vi "Parse Downlink.vi"(7 "CP_DATA IN":u8[](array[numeric]), 8 "error in (no error)":errorcluster, 9 "Parameters":string, 10 "EXID":u32 step=1 format="%06x", 11 "Command":T1) -> (0 "error out":errorcluster, 2 "Downlink":u8[][](array[numeric]) format="%02x")   [LabVIEW 2020]
uses:
  Command List.ctl
  Typedef Command List.ctl
  <vilib>/Utility/miscctls.llb/LVDateTimeRec.ctl
panel:
  in  "Command":T2 items=["Get xPG Status", "xPG Stimulation", "Select Program", "Increment Program Amplitude", "Decrement Program Amplitude", "Get PoP Constants", "Get PPC Constants", "Get Program Names", "Set Pulse Amplitude", "Increment Pulse Amplitude", "Decrement Pulse Amplitude", "Get Pulse Widths", "Set Pulse Widths", "Increment Pulse Width", "Decrement Pulse Width", "Get Program Frequency", "Set Program Frequency", "Increment Program Frequency", "Decrement Program Frequency", "reserved", "Charging Control", "Get xPG Identity", "Set xPG Identity", "Restore Program Defaults", "Get Program Definition", "Set Program Definition", "Get Program Constants", "Set Program Constants", "Get Configurable Device Parameters", "Set Configurable Device Parameters", "Get Pulse Constants", "Set Pulse Constants", "Get Lead Limits", "Set Lead Limits", "Get Channel Calibrations", "Set Channel Calibrations", "reserved", "reserved", "reserved", "reserved", "reserved", "reserved", "Get Stim Asic HV Calibrations", "Set Stim Asic HV Calibrations", "reserved", "reserved", "Get CP Data", "Set CP Data", "Clear Log", "Read Log", "Append Log", "Get Patient Program Runtime", "Set Patient Program Runtimec", "Impedance Measurement", "Enter Storage Mode", "Echo Short", "Echo Long", "Get General Calibration", "Set General Calibration", "Get Trim List", "Set Trim List", "Get Counter", "Set Counter", "Get Test Stimulation", "Set Test Stimulation", "Get Titration Stimulation", "Set Titration Stimulation", "Get Ramp Time", "Set Ramp Time", "Get VBAT", "Set Software Description Block", "Write Memory", "Read Memory", "Reset xPG", "Erase Flash Block", "Write Vectors", "Read Vectors", "Diagnostic Data", "Set Background Impedance", "Get Background Impedence ", "Undefined"]
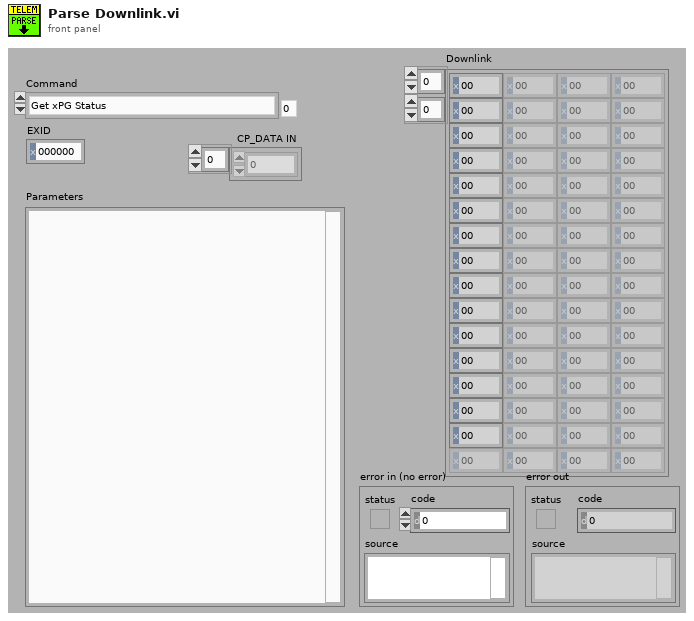
[diagram p1: front panel]
types:
  T1 = typedef "Typedef Command List.ctl" = enum16{"Get xPG Status", "xPG Stimulation", "Select Program", "Increment Program Amplitude", "Decrement Program Amplitude", "Get PoP Constants", "Get PPC Constants", "Get Program Names", "Set Pulse Amplitude", "Increment Pulse Amplitude", "Decrement Pulse Amplitude", "Get Pulse Widths", "Set Pulse Widths", "Increment Pulse Width", "Decrement Pulse Width", "Get Program Frequency", "Set Program Frequency", "Increment Program Frequency", "Decrement Program Frequency", "Inject Event", "Charging Control", "Get xPG Identity", "Set xPG Identity", "Restore Program Defaults", "Get Program Definition", "Set Program Definition", "Get Program Constants", "Set Program Constants", "Get Configurable Device Parameters", "Set Configurable Device Parameters", "Get Pulse Constants", "Set Pulse Constants", "Get Lead Limits", "Set Lead Limits", "Get Channel Calibrations", "Set Channel Calibrations", "<reserved 2>", "<reserved 3>", "<reserved 4>", "<reserved 5>", "<reserved 6>", "<reserved 7>", "Get Stim Asic HV Calibrations", "Set Stim Asic HV Calibrations", "<reserved 8>", "<reserved 9>", "Get CP Data", "Set CP Data", "Clear Log", "Read Log", "Append Log", "Get Patient Program Runtime", "Set Patient Program Runtime", "Impedance Measurement", "Enter Storage Mode", "Echo Short", "Echo Long", "Get General Calibration", "Set General Calibration", "Get Trim List", "Set Trim List", "Get Counter", "Set Counter", "Get Test Stimulation", "Set Test Stimulation", "Get Titration Stimulation", "Set Titration Stimulation", "Get Ramp Time", "Set Ramp Time", "Get VBAT", "Set Software Description Block", "Get Software Description Block", "Write Memory", "Read Memory", "Reset xPG", "Erase Flash Block", "Write Vectors", "Read Vectors", "Diagnostic Data", "Set Background Impedance", "Get Background Impedence ", "Set Test Waveform", "Calibrate Channel", "Get Log Range", "Reserved 0x55", "Reserved 0x56", "MICS Options", "Pair PPC", "Pair POP", "Stop Bootloader", "Tune MICS", "MICS Diagnostics", "Undefined"}
  T2 = typedef "Command List.ctl" = u16
  T3 = enum16{"U8", "U16", "U32", "U64", "I8", "I16", "I32", "I64"}
  T4 = typedef "LVDateTimeRec.ctl" = cluster{"fractional second":dbl, "second":i32, "minute":i32, "hour":i32, "day of month":i32, "month":i32, "year":i32, "day of week":i32, "day of year":i32, "DST":i32}
  T5 = cluster{"CP_DATA IN[0]":u8, "CP_DATA IN[1]":u8, "CP_DATA IN[2]":u8, "CP_DATA IN[3]":u8, "CP_DATA IN[4]":u8, "CP_DATA IN[5]":u8, "CP_DATA IN[6]":u8, "CP_DATA IN[7]":u8, "CP_DATA IN[8]":u8, "CP_DATA IN[9]":u8, "CP_DATA IN[10]":u8, "CP_DATA IN[11]":u8, "CP_DATA IN[12]":u8, "CP_DATA IN[13]":u8, "CP_DATA IN[14]":u8, "CP_DATA IN[15]":u8, "CP_DATA IN[16]":u8, "CP_DATA IN[17]":u8, "CP_DATA IN[18]":u8, "CP_DATA IN[19]":u8, "CP_DATA IN[20]":u8, "CP_DATA IN[21]":u8, "CP_DATA IN[22]":u8, "CP_DATA IN[23]":u8, "CP_DATA IN[24]":u8, "CP_DATA IN[25]":u8, "CP_DATA IN[26]":u8, "CP_DATA IN[27]":u8, "CP_DATA IN[28]":u8, "CP_DATA IN[29]":u8, "CP_DATA IN[30]":u8, "CP_DATA IN[31]":u8, "CP_DATA IN[32]":u8, "CP_DATA IN[33]":u8, "CP_DATA IN[34]":u8, "CP_DATA IN[35]":u8, "CP_DATA IN[36]":u8, "CP_DATA IN[37]":u8, "CP_DATA IN[38]":u8, "CP_DATA IN[39]":u8, "CP_DATA IN[40]":u8, "CP_DATA IN[41]":u8, "CP_DATA IN[42]":u8, "CP_DATA IN[43]":u8, "CP_DATA IN[44]":u8, "CP_DATA IN[45]":u8, "CP_DATA IN[46]":u8, "CP_DATA IN[47]":u8, "CP_DATA IN[48]":u8, "CP_DATA IN[49]":u8, "CP_DATA IN[50]":u8, "CP_DATA IN[51]":u8, "CP_DATA IN[52]":u8, "CP_DATA IN[53]":u8, "CP_DATA IN[54]":u8, "CP_DATA IN[55]":u8, "CP_DATA IN[56]":u8, "CP_DATA IN[57]":u8, "CP_DATA IN[58]":u8, "CP_DATA IN[59]":u8, "CP_DATA IN[60]":u8, "CP_DATA IN[61]":u8, "CP_DATA IN[62]":u8, "CP_DATA IN[63]":u8, "CP_DATA IN[64]":u8, "CP_DATA IN[65]":u8, "CP_DATA IN[66]":u8, "CP_DATA IN[67]":u8, "CP_DATA IN[68]":u8, "CP_DATA IN[69]":u8, "CP_DATA IN[70]":u8, "CP_DATA IN[71]":u8, "CP_DATA IN[72]":u8, "CP_DATA IN[73]":u8, "CP_DATA IN[74]":u8, "CP_DATA IN[75]":u8, "CP_DATA IN[76]":u8, "CP_DATA IN[77]":u8, "CP_DATA IN[78]":u8, "CP_DATA IN[79]":u8, "CP_DATA IN[80]":u8, "CP_DATA IN[81]":u8, "CP_DATA IN[82]":u8, "CP_DATA IN[83]":u8, "CP_DATA IN[84]":u8, "CP_DATA IN[85]":u8, "CP_DATA IN[86]":u8, "CP_DATA IN[87]":u8, "CP_DATA IN[88]":u8, "CP_DATA IN[89]":u8, "CP_DATA IN[90]":u8, "CP_DATA IN[91]":u8, "CP_DATA IN[92]":u8, "CP_DATA IN[93]":u8, "CP_DATA IN[94]":u8, "CP_DATA IN[95]":u8, "CP_DATA IN[96]":u8, "CP_DATA IN[97]":u8, "CP_DATA IN[98]":u8, "CP_DATA IN[99]":u8, "CP_DATA IN[100]":u8, "CP_DATA IN[101]":u8, "CP_DATA IN[102]":u8, "CP_DATA IN[103]":u8, "CP_DATA IN[104]":u8, "CP_DATA IN[105]":u8, "CP_DATA IN[106]":u8, "CP_DATA IN[107]":u8, "CP_DATA IN[108]":u8, "CP_DATA IN[109]":u8, "CP_DATA IN[110]":u8, "CP_DATA IN[111]":u8, "CP_DATA IN[112]":u8, "CP_DATA IN[113]":u8, "CP_DATA IN[114]":u8, "CP_DATA IN[115]":u8, "CP_DATA IN[116]":u8, "CP_DATA IN[117]":u8, "CP_DATA IN[118]":u8, "CP_DATA IN[119]":u8, "CP_DATA IN[120]":u8, "CP_DATA IN[121]":u8, "CP_DATA IN[122]":u8, "CP_DATA IN[123]":u8, "CP_DATA IN[124]":u8, "CP_DATA IN[125]":u8, "CP_DATA IN[126]":u8, "CP_DATA IN[127]":u8, "CP_DATA IN[128]":u8, "CP_DATA IN[129]":u8, "CP_DATA IN[130]":u8, "CP_DATA IN[131]":u8, "CP_DATA IN[132]":u8, "CP_DATA IN[133]":u8, "CP_DATA IN[134]":u8, "CP_DATA IN[135]":u8, "CP_DATA IN[136]":u8, "CP_DATA IN[137]":u8, "CP_DATA IN[138]":u8, "CP_DATA IN[139]":u8, "CP_DATA IN[140]":u8, "CP_DATA IN[141]":u8, "CP_DATA IN[142]":u8, "CP_DATA IN[143]":u8, "CP_DATA IN[144]":u8, "CP_DATA IN[145]":u8, "CP_DATA IN[146]":u8, "CP_DATA IN[147]":u8, "CP_DATA IN[148]":u8, "CP_DATA IN[149]":u8, "CP_DATA IN[150]":u8, "CP_DATA IN[151]":u8, "CP_DATA IN[152]":u8, "CP_DATA IN[153]":u8, "CP_DATA IN[154]":u8, "CP_DATA IN[155]":u8, "CP_DATA IN[156]":u8, "CP_DATA IN[157]":u8, "CP_DATA IN[158]":u8, "CP_DATA IN[159]":u8, "CP_DATA IN[160]":u8, "CP_DATA IN[161]":u8, "CP_DATA IN[162]":u8, "CP_DATA IN[163]":u8, "CP_DATA IN[164]":u8, "CP_DATA IN[165]":u8, "CP_DATA IN[166]":u8, "CP_DATA IN[167]":u8, "CP_DATA IN[168]":u8, "CP_DATA IN[169]":u8, "CP_DATA IN[170]":u8, "CP_DATA IN[171]":u8, "CP_DATA IN[172]":u8, "CP_DATA IN[173]":u8, "CP_DATA IN[174]":u8, "CP_DATA IN[175]":u8, "CP_DATA IN[176]":u8, "CP_DATA IN[177]":u8, "CP_DATA IN[178]":u8, "CP_DATA IN[179]":u8, "CP_DATA IN[180]":u8, "CP_DATA IN[181]":u8, "CP_DATA IN[182]":u8, "CP_DATA IN[183]":u8, "CP_DATA IN[184]":u8, "CP_DATA IN[185]":u8, "CP_DATA IN[186]":u8, "CP_DATA IN[187]":u8, "CP_DATA IN[188]":u8, "CP_DATA IN[189]":u8, "CP_DATA IN[190]":u8, "CP_DATA IN[191]":u8, "CP_DATA IN[192]":u8, "CP_DATA IN[193]":u8, "CP_DATA IN[194]":u8, "CP_DATA IN[195]":u8, "CP_DATA IN[196]":u8, "CP_DATA IN[197]":u8, "CP_DATA IN[198]":u8, "CP_DATA IN[199]":u8, "CP_DATA IN[200]":u8, "CP_DATA IN[201]":u8, "CP_DATA IN[202]":u8, "CP_DATA IN[203]":u8, "CP_DATA IN[204]":u8, "CP_DATA IN[205]":u8, "CP_DATA IN[206]":u8, "CP_DATA IN[207]":u8, "CP_DATA IN[208]":u8, "CP_DATA IN[209]":u8, "CP_DATA IN[210]":u8, "CP_DATA IN[211]":u8, "CP_DATA IN[212]":u8, "CP_DATA IN[213]":u8, "CP_DATA IN[214]":u8, "CP_DATA IN[215]":u8, "CP_DATA IN[216]":u8, "CP_DATA IN[217]":u8, "CP_DATA IN[218]":u8, "CP_DATA IN[219]":u8, "CP_DATA IN[220]":u8, "CP_DATA IN[221]":u8, "CP_DATA IN[222]":u8, "CP_DATA IN[223]":u8, "CP_DATA IN[224]":u8, "CP_DATA IN[225]":u8, "CP_DATA IN[226]":u8, "CP_DATA IN[227]":u8, "CP_DATA IN[228]":u8, "CP_DATA IN[229]":u8, "CP_DATA IN[230]":u8, "CP_DATA IN[231]":u8, "CP_DATA IN[232]":u8, "CP_DATA IN[233]":u8, "CP_DATA IN[234]":u8, "CP_DATA IN[235]":u8, "CP_DATA IN[236]":u8, "CP_DATA IN[237]":u8, "CP_DATA IN[238]":u8, "CP_DATA IN[239]":u8, "CP_DATA IN[240]":u8, "CP_DATA IN[241]":u8, "CP_DATA IN[242]":u8, "CP_DATA IN[243]":u8, "CP_DATA IN[244]":u8, "CP_DATA IN[245]":u8, "CP_DATA IN[246]":u8, "CP_DATA IN[247]":u8, "CP_DATA IN[248]":u8, "CP_DATA IN[249]":u8, "CP_DATA IN[250]":u8, "CP_DATA IN[251]":u8, "CP_DATA IN[252]":u8, "CP_DATA IN[253]":u8, "CP_DATA IN[254]":u8, "CP_DATA IN[255]":u8}
  T6 = cluster{"Byte Data[0]":u8, "Byte Data[1]":u8, "Byte Data[2]":u8, "Byte Data[3]":u8, "Byte Data[4]":u8, "Byte Data[5]":u8, "Byte Data[6]":u8, "Byte Data[7]":u8, "Byte Data[8]":u8}
  T7 = cluster{"DATA[0]":u8, "DATA[1]":u8, "DATA[2]":u8, "DATA[3]":u8, "DATA[4]":u8, "DATA[5]":u8, "DATA[6]":u8, "DATA[7]":u8, "DATA[8]":u8, "DATA[9]":u8, "DATA[10]":u8, "DATA[11]":u8, "DATA[12]":u8, "DATA[13]":u8, "DATA[14]":u8}
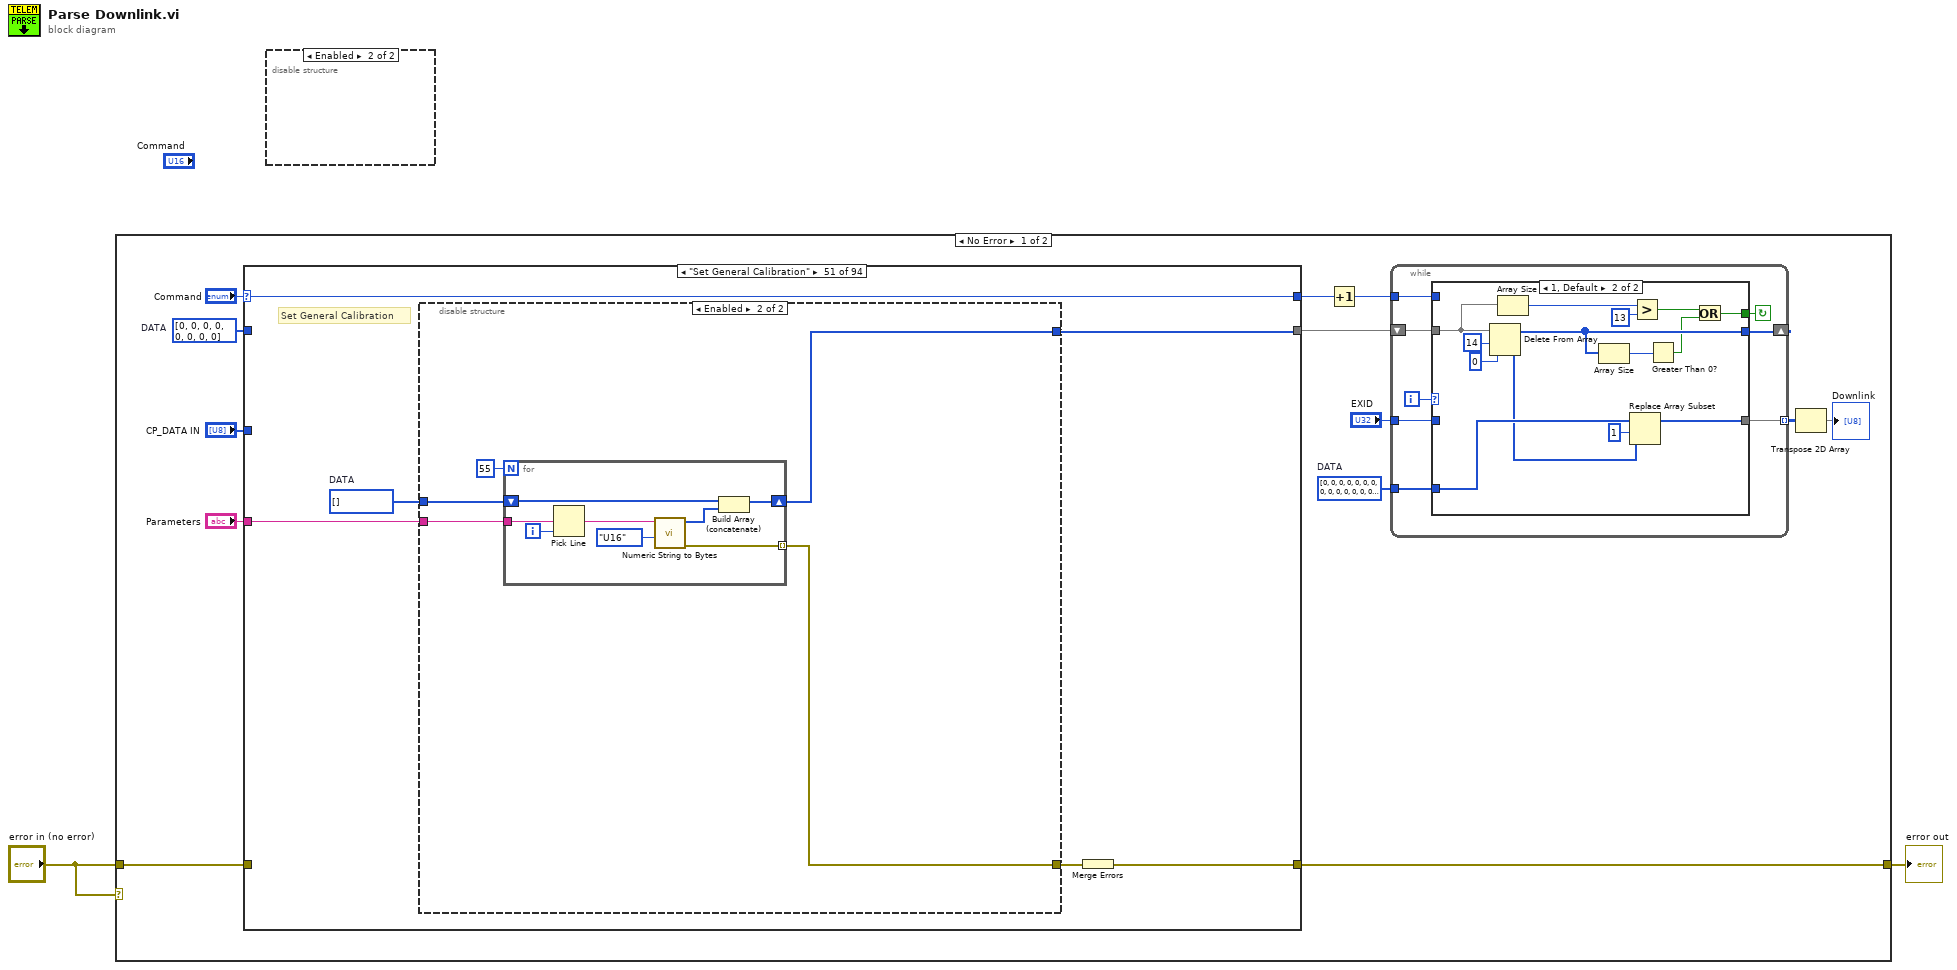
[diagram p0: block diagram]
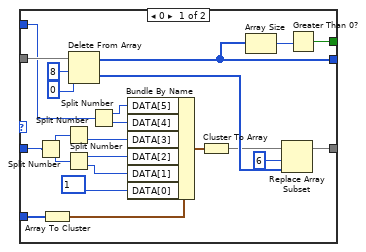
[diagram p3: hidden frame]
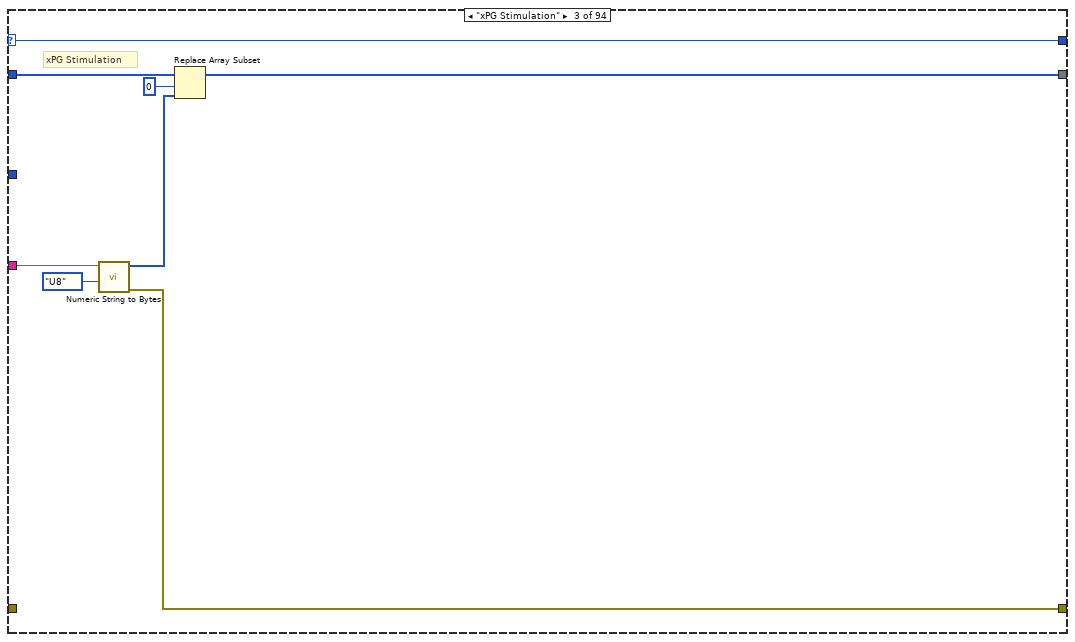
[diagram p6: hidden frame]
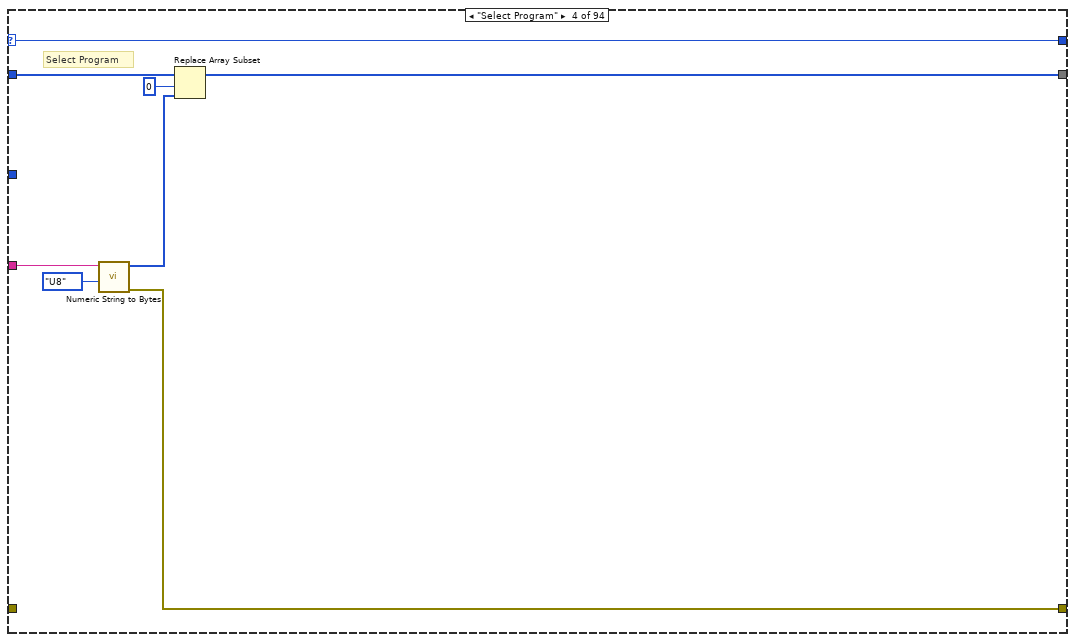
[diagram p7: hidden frame]
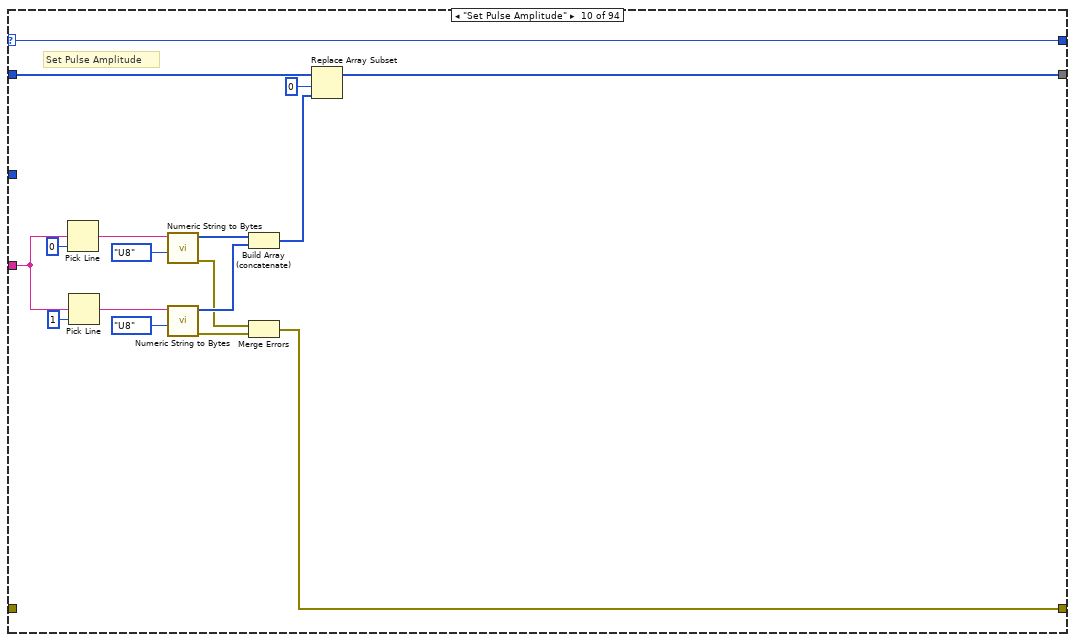
[diagram p13: hidden frame]
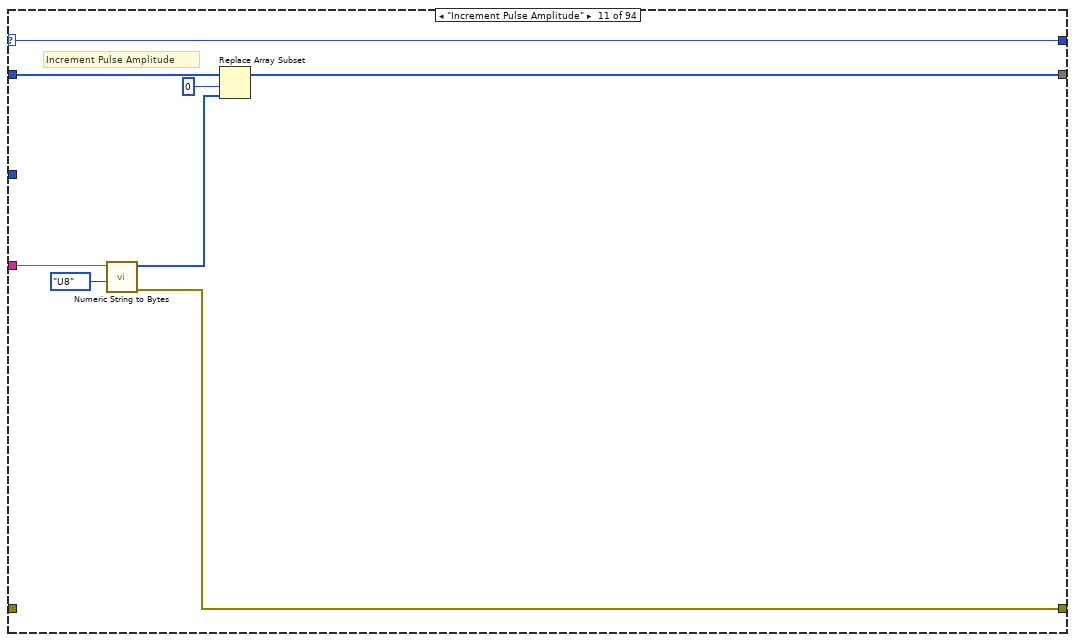
[diagram p14: hidden frame]
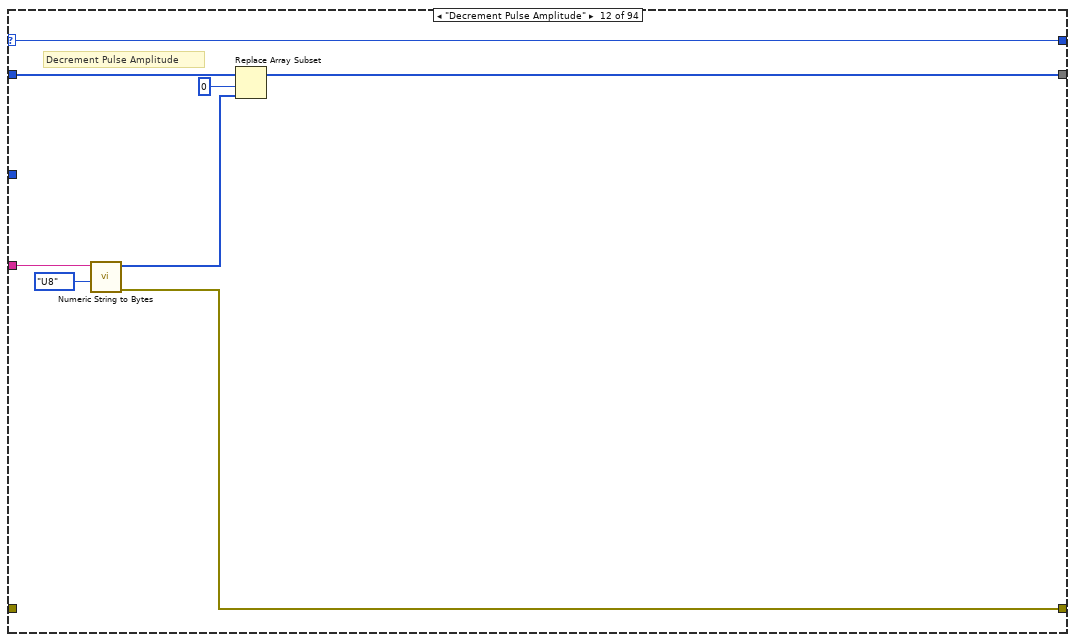
[diagram p15: hidden frame]
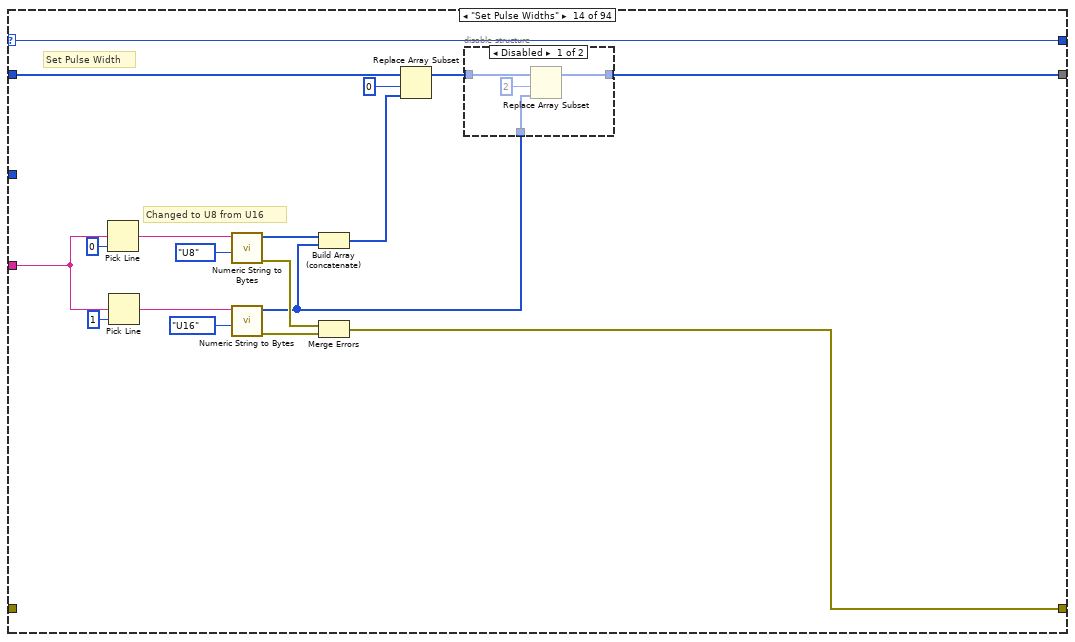
[diagram p17: hidden frame]
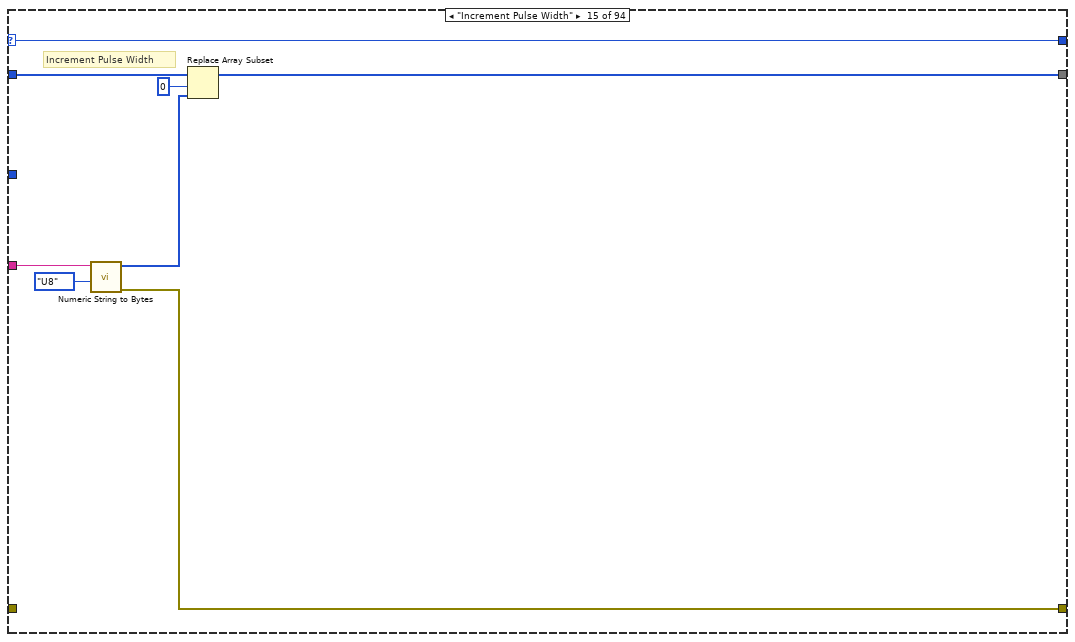
[diagram p19: hidden frame]
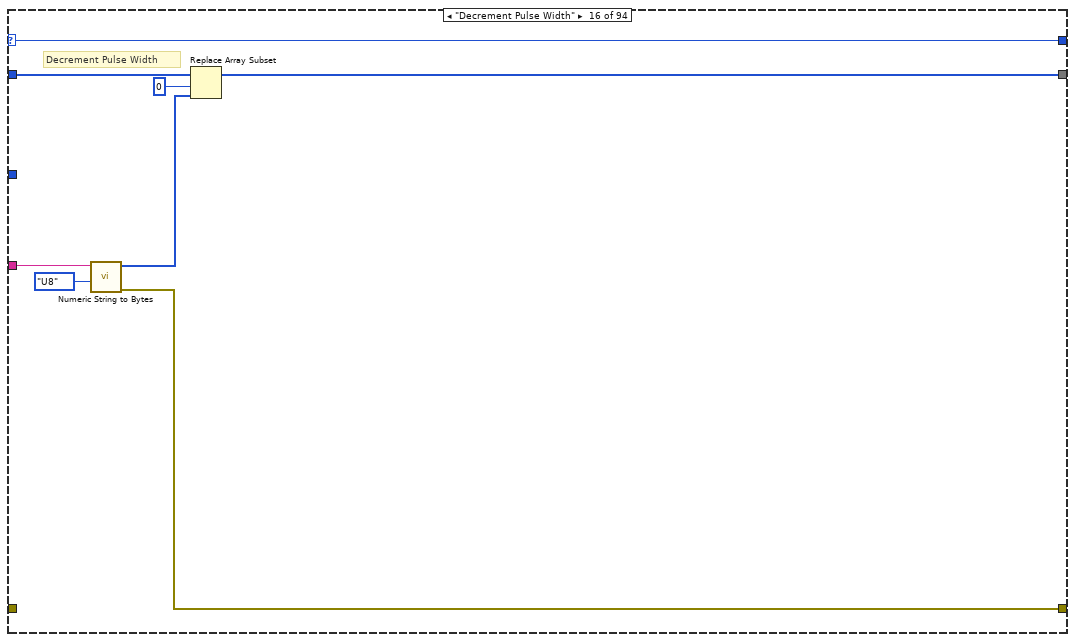
[diagram p20: hidden frame]
diagram:
  n1 = case shown="No Error" "error in (no error)" {
    tunnel: "error in (no error)" -> [w8 w1303]
    tunnel: [w7 w1303] -> w2
    frame No Error {
      w9 = u8[] [0, 0, 0, 0, 0, 0, 0, 0]  # DATA
      w10 = u8[] [0, 0, 0, 0, 0, 0, 0, 0, 0, 0, 0, 0, 0, 0, 0]  # DATA
      n2 = case shown="\"Set General Calibration\"" "Command" {
        selector: "Command" -> [w63 w66 w74 w82 w85 w88 w91 w94 w97 w114 w122 w130 w133 w151 w164 w172 w175 w183 w186 w189 w192 w195 w221 w237 w245 w252 w395 w409 w422 w497 w512 w531 w542 w549 w565 w578 w590 w597 w613 w625 w633 w651 w689 w697 w715 w738 w741 w747 w753 w756 w762 w864 w866 w956 w975 w978 w1002 w1059 w1078 w1110 w1118 w1121 w1124 w1127 w1153 w1175 w1178 w1181 w1184 w1187 w1204 w1218 w1232 w1235 w1237 w1240 w1251 w1253 w1256 w1259 w1262 w1265 w1268 w1271 w1274 w1277 w1280 w1283 w1286 w1289 w1292 w1295 w1298 w1301]
        tunnel: "Parameters" -> [_ _ w72 w80 _ _ _ _ _ w113 w120 w128 _ w139 w162 w170 _ w181 _ _ _ _ w219 w235 w243 w247 _ w397 _ w427 _ w518 _ w546 w560 w567 _ w594 w611 w620 w631 w635 w654 w695 w698 w716 _ _ _ _ w758 w859 w868 w954 w959 _ w984 _ w1069 _ w1115 _ _ _ w1143 w1170 _ _ _ _ w1200 w1208 w1222 _ _ _ w1244 _ _ _ _ _ _ _ _ _ _ _ _ _ _ _ _ _]
        tunnel: [w63 w66 w74 w82 w85 w88 w91 w94 w97 w114 w122 w130 w133 w151 w164 w172 w175 w183 w186 w189 w192 w195 w221 w237 w245 w252 w395 w409 w422 w497 w512 w531 w542 w549 w565 w578 w590 w597 w613 w625 w633 w651 w689 w697 w715 w738 w741 w747 w753 w756 w762 w864 w866 w956 w975 w978 w1002 w1059 w1078 w1110 w1118 w1121 w1124 w1127 w1153 w1175 w1178 w1181 w1184 w1187 w1204 w1218 w1232 w1235 w1237 w1240 w1251 w1253 w1256 w1259 w1262 w1265 w1268 w1271 w1274 w1277 w1280 w1283 w1286 w1289 w1292 w1295 w1298 w1301] -> w15
        tunnel: [w62 w65 w70 w78 w84 w87 w90 w93 w96 w106 w118 w126 w132 w137 w160 w168 w174 w179 w185 w188 w191 w194 w207 w233 w241 w248 w394 w407 w421 w494 w511 w528 w541 w544 w558 w570 w589 w592 w609 w619 w629 w649 w687 w693 w713 w736 w740 w743 w749 w755 w759 w857 w867 w952 w973 w976 w981 w1057 w1064 w1108 w1112 w1119 w1122 w1125 w1133 w1159 w1176 w1179 w1182 w1185 w1188 w1213 w1227 w1234 w1236 w1239 w1245 w1252 w1255 w1258 w1261 w1264 w1267 w1270 w1273 w1276 w1279 w1282 w1285 w1288 w1291 w1294 w1297 w1300] -> w13
        tunnel: w9 -> [w62 w65 w73 w81 w84 w87 w90 w93 w96 w105 w121 w129 w132 w144 w163 w171 w174 w182 w185 w188 w191 w194 _ w236 w244 _ w394 _ w421 _ w511 _ w541 _ w559 _ w589 _ w612 _ w632 w650 w688 w696 w714 w737 w740 _ _ w755 _ w860 _ w955 w974 w976 _ w1057 _ w1108 w1114 w1119 w1122 w1125 w1131 w1160 w1176 w1179 w1182 w1185 w1191 _ _ w1234 w1236 w1239 w1246 w1252 w1255 w1258 w1261 w1264 w1267 w1270 w1273 w1276 w1279 w1282 w1285 w1288 w1291 w1294 w1297 w1300]
        tunnel: w8 -> [w61 w64 _ _ w83 w86 w89 w92 w95 _ _ _ w131 _ _ _ w173 _ w184 w187 w190 w193 _ _ _ w250 w393 _ w420 _ w510 _ w540 _ _ _ w588 _ _ _ _ _ _ _ _ _ w739 w742 w748 w754 _ _ _ _ _ w977 _ w1058 _ w1109 _ w1120 w1123 w1126 _ _ w1177 w1180 w1183 w1186 _ _ _ w1233 w1238 w1241 _ w1254 w1257 w1260 w1263 w1266 w1269 w1272 w1275 w1278 w1281 w1284 w1287 w1290 w1293 w1296 w1299 w1302]
        tunnel: [w61 w64 w71 w79 w83 w86 w89 w92 w95 w98 w119 w127 w131 w140 w161 w169 w173 w180 w184 w187 w190 w193 w197 w234 w242 w249 w393 w400 w420 w495 w510 w527 w540 w547 w561 w576 w588 w595 w610 w624 w630 w636 w673 w694 w699 w722 w739 w742 w748 w754 w760 w858 w865 w953 w960 w977 w982 w1058 w1060 w1109 w1111 w1120 w1123 w1126 w1142 w1161 w1177 w1180 w1183 w1186 w1192 w1205 w1219 w1233 w1238 w1241 w1242 w1254 w1257 w1260 w1263 w1266 w1269 w1272 w1275 w1278 w1281 w1284 w1287 w1290 w1293 w1296 w1299 w1302] -> w7
        tunnel: "CP_DATA IN" -> [_ _ _ _ _ _ _ _ _ _ _ _ _ _ _ _ _ _ _ _ _ _ _ _ _ _ _ _ _ _ _ _ _ _ _ _ _ _ _ w616 _ _ _ _ _ _ _ w746 w752 _ _ _ _ _ _ _ _ _ _ _ _ _ _ _ w1139 _ _ _ _ _ _ _ _ _ _ _ _ _ _ _ _ _ _ _ _ _ _ _ _ _ _ _ _ _]
        frame Default {
          # "NULL"
        }
        frame "Get xPG Status" {
          # "Get xPG Status"
        }
        frame "xPG Stimulation" {
          # "xPG Stimulation"
          n3 = call "Numeric String to Bytes.vi"("Type"=T3."U8", "String"=w72) -> ("error out"=w71:errorcluster, "Byte Data"=w68:u8[])  [unwired: 8 in]
          n4 = Replace Array Subset(array=w73, new element=w68, index=0) -> (w70:u8[])
        }
        frame "Select Program" {
          # "Select Program"
          n5 = call "Numeric String to Bytes.vi"("Type"=T3."U8", "String"=w80) -> ("error out"=w79:errorcluster, "Byte Data"=w76:u8[])  [unwired: 8 in]
          n6 = Replace Array Subset(array=w81, new element=w76, index=0) -> (w78:u8[])
        }
        frame "Increment Program Amplitude" {
          # "Increment Program Amplitude"
        }
        frame "Decrement Program Amplitude" {
          # "Decrement Program Amplitude"
        }
        frame "Get PoP Constants" {
          # "Get PoP Constants"
        }
        frame "Get PPC Constants" {
          # "Get PPC Constants"
        }
        frame "Get Program Names" {
          # "Get Program Names"
        }
        frame "Set Pulse Amplitude" {
          # "Set Pulse Amplitude"
          n7 = Pick Line(multi-line string=w113, line index=0) -> (output string=w107:string)  [unwired: 1 in]
          n8 = Pick Line(multi-line string=w113, line index=1) -> (output string=w108:string)  [unwired: 1 in]
          n9 = call "Numeric String to Bytes.vi"("Type"=T3."U8", "String"=w107) -> ("error out"=w100:errorcluster, "Byte Data"=w104:u8[])  [unwired: 8 in]
          n10 = call "Numeric String to Bytes.vi"("Type"=T3."U8", "String"=w108) -> ("error out"=w99:errorcluster, "Byte Data"=w103:u8[])  [unwired: 8 in]
          n11 = Build Array (concatenate)(w104, w103) -> (w101:u8[])
          n12 = Merge Errors(w100, w99) -> (w98:errorcluster)
          n13 = Replace Array Subset(array=w105, new element=w101, index=0) -> (w106:u8[])
        }
        frame "Increment Pulse Amplitude" {
          # "Increment Pulse Amplitude"
          n14 = call "Numeric String to Bytes.vi"("Type"=T3."U8", "String"=w120) -> ("error out"=w119:errorcluster, "Byte Data"=w116:u8[])  [unwired: 8 in]
          n15 = Replace Array Subset(array=w121, new element=w116, index=0) -> (w118:u8[])
        }
        frame "Decrement Pulse Amplitude" {
          # "Decrement Pulse Amplitude"
          n16 = call "Numeric String to Bytes.vi"("Type"=T3."U8", "String"=w128) -> ("error out"=w127:errorcluster, "Byte Data"=w124:u8[])  [unwired: 8 in]
          n17 = Replace Array Subset(array=w129, new element=w124, index=0) -> (w126:u8[])
        }
        frame "Get Pulse Widths" {
          # "Get Pulse Widths"
        }
        frame "Set Pulse Widths" {
          # "Changed to U8 from U16"
          # "Set Pulse Width"
          n18 = Pick Line(multi-line string=w139, line index=0) -> (output string=w145:string)  [unwired: 1 in]
          n19 = Pick Line(multi-line string=w139, line index=1) -> (output string=w146:string)  [unwired: 1 in]
          n20 = call "Numeric String to Bytes.vi"("Type"=T3."U8", "String"=w145) -> ("error out"=w142:errorcluster, "Byte Data"=w136:u8[])  [unwired: 8 in]
          n21 = call "Numeric String to Bytes.vi"("Type"=T3."U16", "String"=w146) -> ("error out"=w141:errorcluster, "Byte Data"=w135:u8[])  [unwired: 8 in]
          n22 = Build Array (concatenate)(w136, w135) -> (w134:u8[])
          n23 = Merge Errors(w142, w141) -> (w140:errorcluster)
          n24 = Replace Array Subset(array=w144, new element=w134, index=0) -> (w138:u8[])
          n25 = disable-structure shown="Disabled" {
            disable-tunnel: w135 -> [w154 _]
            disable-tunnel: w138 -> [w153 w156]
            disable-tunnel: [w152 w156] -> w137
            frame Disabled {
              n26 = Replace Array Subset(array=w153, new element=w154, index=2) -> (w152:u8[])
            }
            frame Enabled {
            }
          }
        }
        frame "Increment Pulse Width" {
          # "Increment Pulse Width"
          n27 = call "Numeric String to Bytes.vi"("Type"=T3."U8", "String"=w162) -> ("error out"=w161:errorcluster, "Byte Data"=w158:u8[])  [unwired: 8 in]
          n28 = Replace Array Subset(array=w163, new element=w158, index=0) -> (w160:u8[])
        }
        frame "Decrement Pulse Width" {
          # "Decrement Pulse Width"
          n29 = call "Numeric String to Bytes.vi"("Type"=T3."U8", "String"=w170) -> ("error out"=w169:errorcluster, "Byte Data"=w166:u8[])  [unwired: 8 in]
          n30 = Replace Array Subset(array=w171, new element=w166, index=0) -> (w168:u8[])
        }
        frame "Get Program Frequency" {
          # "Get Program Frequency"
        }
        frame "Set Program Frequency" {
          # "Set Program Frequency"
          n31 = call "Numeric String to Bytes.vi"("Type"=T3."U8", "String"=w181) -> ("error out"=w180:errorcluster, "Byte Data"=w177:u8[])  [unwired: 8 in]
          n32 = Replace Array Subset(array=w182, new element=w177, index=0) -> (w179:u8[])
        }
        frame "Increment Program Frequency" {
          # "Increment Program Frequency"
        }
        frame "Decrement Program Frequency" {
          # "Decrement Program Frequency"
        }
        frame "Charging Control" {
          # "Charging Control"
        }
        frame "Get xPG Identity" {
          # "Get xPG Identity"
        }
        frame "Set xPG Identity" {
          w196 = u8[] [0, 0, 0, 0]  # DATA
          w213 = u8[] [0, 0, 0, 0, 0, 0, 0, 0, 0, 0, 0, 0, 0, 0, 0, 0, 0, 0, 0, 0]  # DATA
          w214 = u8[] [0, 0, 0, 0, 0, 0, 0, 0, 0, 0]  # DATA
          # "Set xPG Identity"
          n33 = Pick Line(multi-line string=w219, line index=4) -> (output string=w203:string)  [unwired: 1 in]
          n34 = Pick Line(multi-line string=w219, line index=5) -> (output string=w200:string)  [unwired: 1 in]
          n35 = for {
            N: 4 -> [_]
            tunnel: w219 -> [w229]
            shift-right: [w225] -> w210
            shift-left: w196 -> [w226]
            tunnel: [w224] -> w198 mode=indexing
            i -> [w222]
            n36 = Pick Line(multi-line string=w229, line index=w222) -> (output string=w228:string)  [unwired: 1 in]
            n37 = call "Numeric String to Bytes.vi"("Type"=T3."U8", "String"=w228) -> ("error out"=w224:errorcluster, "Byte Data"=w223:u8[])  [unwired: 8 in]
            n38 = Replace Array Subset(array=w226, new element=w223, index=w222) -> (w225:u8[])
          }
          n39 = Match Pattern(string=w203, regular expression="=") -> (after substring=w202:string)  [unwired: 1 in, 3 out]
          n40 = Match Pattern(string=w200, regular expression="=") -> (after substring=w199:string)  [unwired: 1 in, 3 out]
          n41 = call <vilib>:"Trim Whitespace.vi"("string"=w202) -> ("trimmed string"=w216:string)  [unwired: 1 in]
          n42 = call <vilib>:"Trim Whitespace.vi"("string"=w199) -> ("trimmed string"=w215:string)  [unwired: 1 in]
          n43 = String To Byte Array(string=w216) -> (unsigned byte array=w211:u8[])
          n44 = String To Byte Array(string=w215) -> (unsigned byte array=w212:u8[])
          n45 = Replace Array Subset(array=w214, new element=w211, index=0) -> (w209:u8[])
          n46 = Replace Array Subset(array=w213, new element=w212, index=0) -> (w208:u8[])
          n47 = Build Array (concatenate)(w210, w209, w208) -> (w207:u8[])
          n48 = Merge Errors(w198) -> (w197:errorcluster)
        }
        frame "Restore Program Defaults" {
          # "Restore Program Defaults"
          n49 = call "Numeric String to Bytes.vi"("Type"=T3."U16", "String"=w235) -> ("error out"=w234:errorcluster, "Byte Data"=w231:u8[])  [unwired: 8 in]
          n50 = Replace Array Subset(array=w236, new element=w231, index=0) -> (w233:u8[])
        }
        frame "Get Program Definition" {
          # "Get Program Definition"
          n51 = call "Numeric String to Bytes.vi"("Type"=T3."U8", "String"=w243) -> ("error out"=w242:errorcluster, "Byte Data"=w239:u8[])  [unwired: 8 in]
          n52 = Replace Array Subset(array=w244, new element=w239, index=0) -> (w241:u8[])
        }
        frame "Set Program Definition" {
          w251 = u8[] []  # DATA
          # "Set Program Definition"
          n53 = while {
            shift-right: [w256] -> w248
            shift-left: w251 -> [w257]
            shift-right: [w262] -> w249
            shift-left: w250 -> [w263]
            tunnel: w247 -> [w255]
            shift-right: [w253] -> _
            shift-left: 0 -> [w254]
            i -> [w258]
            stop <- w259 stop-if-true
            n54 = case shown="1, Default" w258 {
              tunnel: w263 -> [w275 w327]
              tunnel: [w274 w326] -> w262
              tunnel: [FALSE ("status") TRUE ("status")] -> w260
              tunnel: w257 -> [w288 w330]
              tunnel: [w287 w329] -> w256
              tunnel: w255 -> [w290 w324]
              tunnel: w254 -> [_ w325]
              tunnel: [14 ("line index") w322] -> w253
              frame 0 {
                w304 = u8[] [0, 0, 0, 0, 0, 0, 0, 0, 0, 0, 0, 0, 0, 0, 0, 0]  # DATA
                # "Changed to U8 from U16"
                n55 = Pick Line(multi-line string=w290, line index=3) -> (output string=w271:string)  [unwired: 1 in]
                n56 = Pick Line(multi-line string=w290, line index=0) -> (output string=w297:string)  [unwired: 1 in]
                n57 = Pick Line(multi-line string=w290, line index=1) -> (output string=w298:string)  [unwired: 1 in]
                n58 = Pick Line(multi-line string=w290, line index=2) -> (output string=w299:string)  [unwired: 1 in]
                n59 = Pick Line(multi-line string=w290, line index=12) -> (output string=w294:string)  [unwired: 1 in]
                n60 = Pick Line(multi-line string=w290, line index=13) -> (output string=w291:string)  [unwired: 1 in]
                n61 = for {
                  N: 8 -> [_]
                  tunnel: w290 -> [w321]
                  shift-right: [w313] -> w284
                  shift-left: w288 -> [w314]
                  tunnel: [w312] -> w269 mode=indexing
                  i -> [w319]
                  n62 = Add(x=4 ("line index"), y=w319) -> (x+y=w318:i32)
                  n63 = Pick Line(multi-line string=w321, line index=w318) -> (output string=w316:string)  [unwired: 1 in]
                  n64 = call "Numeric String to Bytes.vi"("Type"=T3."U8", "String"=w316) -> ("error out"=w312:errorcluster, "Byte Data"=w315:u8[])  [unwired: 8 in]
                  n65 = Build Array (concatenate)(w314, w315) -> (w313:u8[])
                }
                n66 = Match Pattern(string=w271, regular expression="=") -> (after substring=w270:string)  [unwired: 1 in, 3 out]
                n67 = call <vilib>:"Trim Whitespace.vi"("string"=w270) -> ("trimmed string"=w307:string)  [unwired: 1 in]
                n68 = call "Numeric String to Bytes.vi"("Type"=T3."U8", "String"=w297) -> ("error out"=w280:errorcluster, "Byte Data"=w286:u8[])  [unwired: 8 in]
                n69 = call "Numeric String to Bytes.vi"("Type"=T3."U8", "String"=w298) -> ("error out"=w279:errorcluster, "Byte Data"=w268:u8[])  [unwired: 8 in]
                n70 = call "Numeric String to Bytes.vi"("Type"=T3."U8", "String"=w299) -> ("error out"=w278:errorcluster, "Byte Data"=w285:u8[])  [unwired: 8 in]
                n71 = call "Numeric String to Bytes.vi"("Type"=T3."U8", "String"=w294) -> ("error out"=w277:errorcluster, "Byte Data"=w283:u8[])  [unwired: 8 in]
                n72 = call "Numeric String to Bytes.vi"("Type"=T3."U8", "String"=w291) -> ("error out"=w276:errorcluster, "Byte Data"=w282:u8[])  [unwired: 8 in]
                n73 = String To Byte Array(string=w307) -> (unsigned byte array=w306:u8[])
                n74 = Replace Array Subset(array=w304, new element=w306, index=0) -> (w264:u8[])
                n75 = Split 1D Array(array=w264, index=16) -> (first subarray=w265:u8[])  [unwired: 1 out]
                n76 = Build Array (concatenate)(w288, w286, u8[] [0] ("array"), w268, w285, w265, w284, w283, w282) -> (w287:u8[])
                n77 = Build Array (concatenate)(w280, w279, w278, w269, w277, w276, w275) -> (w273:errorcluster[])
                n78 = Merge Errors(w273) -> (w274:errorcluster)
              }
              frame 1, Default {
                n79 = for {
                  N: 4 -> [_]
                  shift-right: [w348] -> w329
                  shift-left: w330 -> [w365]
                  shift-right: [w350] -> w326
                  shift-left: w327 -> [w357]
                  tunnel: w324 -> [w342]
                  shift-right: [w336] -> w322
                  shift-left: w325 -> [w343]
                  w341 = u8[] []  # DATA
                  w334 = u8[] [0, 0, 0, 0, 0, 0, 0, 0, 0, 0, 0, 0, 0, 0, 0, 0]  # DATA
                  n80 = Increment(x=w343) -> (x+1=w337:i32)
                  n81 = Increment(x=w337) -> (x+1=w368:i32)
                  n82 = Pick Line(multi-line string=w342, line index=w343) -> (output string=w340:string)  [unwired: 1 in]
                  n83 = Pick Line(multi-line string=w342, line index=w337) -> (output string=w380:string)  [unwired: 1 in]
                  n84 = Increment(x=w368) -> (x+1=w369:i32)
                  n85 = Pick Line(multi-line string=w342, line index=w368) -> (output string=w381:string)  [unwired: 1 in]
                  n86 = Match Pattern(string=w340, regular expression="=") -> (after substring=w339:string)  [unwired: 1 in, 3 out]
                  n87 = Increment(x=w369) -> (x+1=w370:i32)
                  n88 = Pick Line(multi-line string=w342, line index=w369) -> (output string=w374:string)  [unwired: 1 in]
                  n89 = Increment(x=w370) -> (x+1=w371:i32)
                  n90 = Pick Line(multi-line string=w342, line index=w370) -> (output string=w375:string)  [unwired: 1 in]
                  n91 = call <vilib>:"Trim Whitespace.vi"("string"=w339) -> ("trimmed string"=w346:string)  [unwired: 1 in]
                  n92 = Increment(x=w371) -> (x+1=w367:i32)
                  n93 = Pick Line(multi-line string=w342, line index=w371) -> (output string=w376:string)  [unwired: 1 in]
                  n94 = Increment(x=w367) -> (x+1=w366:i32)
                  n95 = String To Byte Array(string=w346) -> (unsigned byte array=w345:u8[])
                  n96 = Pick Line(multi-line string=w342, line index=w367) -> (output string=w372:string)  [unwired: 1 in]
                  n97 = for {
                    N: 26 -> [_]
                    tunnel: w342 -> [w392]
                    shift-right: [w387] -> w358
                    shift-left: w341 -> [w388]
                    shift-right: [w385] -> w336
                    shift-left: w366 -> [w386]
                    tunnel: [w384] -> w335 mode=indexing
                    n98 = Pick Line(multi-line string=w392, line index=w386) -> (output string=w390:string)  [unwired: 1 in]
                    n99 = Increment(x=w386) -> (x+1=w385:i32)
                    n100 = call "Numeric String to Bytes.vi"("Type"=T3."I8", "String"=w390) -> ("error out"=w384:errorcluster, "Byte Data"=w389:u8[])  [unwired: 8 in]
                    n101 = Build Array (concatenate)(w388, w389) -> (w387:u8[])
                  }
                  n102 = Replace Array Subset(array=w334, new element=w345, index=0) -> (w332:u8[])
                  n103 = call "Numeric String to Bytes.vi"("Type"=T3."U16", "String"=w380) -> ("error out"=w356:errorcluster, "Byte Data"=w364:u8[])  [unwired: 8 in]
                  n104 = call "Numeric String to Bytes.vi"("Type"=T3."U16", "String"=w381) -> ("error out"=w355:errorcluster, "Byte Data"=w363:u8[])  [unwired: 8 in]
                  n105 = call "Numeric String to Bytes.vi"("Type"=T3."I16", "String"=w374) -> ("error out"=w354:errorcluster, "Byte Data"=w362:u8[])  [unwired: 8 in]
                  n106 = call "Numeric String to Bytes.vi"("Type"=T3."U16", "String"=w375) -> ("error out"=w353:errorcluster, "Byte Data"=w361:u8[])  [unwired: 8 in]
                  n107 = call "Numeric String to Bytes.vi"("Type"=T3."U16", "String"=w376) -> ("error out"=w352:errorcluster, "Byte Data"=w360:u8[])  [unwired: 8 in]
                  n108 = call "Numeric String to Bytes.vi"("Type"=T3."U16", "String"=w372) -> ("error out"=w351:errorcluster, "Byte Data"=w359:u8[])  [unwired: 8 in]
                  n109 = Split 1D Array(array=w332, index=16) -> (first subarray=w331:u8[])  [unwired: 1 out]
                  n110 = Build Array (concatenate)(w365, w331, w364, w363, w362, w361, w360, w359, w358) -> (w348:u8[])
                  n111 = Build Array (concatenate)(w357, w356, w355, w354, w353, w352, w351, w335) -> (w349:errorcluster[])
                  n112 = Merge Errors(w349) -> (w350:errorcluster)
                }
              }
            }
            n113 = Unbundle By Name(w262) -> ("status"=w261:bool)
            n114 = Or(x=w260, y=w261) -> (x .or. y?=w259:bool)
          }
        }
        frame "Get Program Constants" {
          # "Get Program Constants"
        }
        frame "Set Program Constants" {
          w406 = u8[] []  # DATA
          # "Set Program Constants"
          n115 = Pick Line(multi-line string=w397, line index=0) -> (output string=w403:string)  [unwired: 1 in]
          n116 = for {
            N: 64 -> [_]
            tunnel: w397 -> [w419]
            shift-right: [w412] -> w405
            shift-left: w406 -> [w413]
            tunnel: 1 -> [w414]
            tunnel: [w410] -> w399 mode=indexing
            i -> [w416]
            n117 = Add(x=w414, y=w416) -> (x+y=w415:i32)
            n118 = Pick Line(multi-line string=w419, line index=w415) -> (output string=w418:string)  [unwired: 1 in]
            n119 = call "Numeric String to Bytes.vi"("Type"=T3."U16", "String"=w418) -> ("error out"=w410:errorcluster, "Byte Data"=w411:u8[])  [unwired: 8 in]
            n120 = Build Array (concatenate)(w413, w411) -> (w412:u8[])
          }
          n121 = call "Numeric String to Bytes.vi"("Type"=T3."U16", "String"=w403) -> ("error out"=w398:errorcluster, "Byte Data"=w401:u8[])  [unwired: 8 in]
          n122 = Build Array (concatenate)(w401, w405) -> (w407:u8[])
          n123 = Merge Errors(w398, w399) -> (w400:errorcluster)
        }
        frame "Get Configurable Device Parameters" {
          # "Get Configurable Device Parameters"
        }
        frame "Set Configurable Device Parameters" {
          w423 = u8[] [0] ("array")
          w445 = 0
          w489 = u8[] [0, 0, 0, 0, 0, 0, 0, 0, 0, 0, 0, 0, 0, 0, 0, 0, 0, 0, 0, 0, 0, 0, 0, 0, 0, 0, 0, 0, 0, 0]  # DATA
          w496 = u8[] []  # DATA
          # "Changed to U8 from U16"
          # "Set Configurable Device Parameters"
          n124 = Pick Line(multi-line string=w427, line index=17) -> (output string=w425:string)  [unwired: 1 in]
          n125 = Match Pattern(string=w425, regular expression="=") -> (after substring=w424:string)  [unwired: 1 in, 3 out]
          n126 = Scan From String(format string="%d/%d/%d %d=%d=%d %s", input string=w424) -> (error out=w443:errorcluster, output 1=w453:i32, output 2=w452:i32, output 3=w451:i32, output 4=w450:i32, output 5=w449:i32, output 6=w448:i32, output 7=w454:string)  [unwired: 9 in, 2 out]
          n127 = case shown="\"PM\"" w454 {
            tunnel: w450 -> [w498 w500]
            tunnel: [w498 w499] -> w447
            frame Default {
            }
            frame "PM" {
              n128 = Add(x=w500, y=12) -> (x+y=w499:i32)
            }
          }
          n129 = for {
            N: 12 -> [_]
            tunnel: [w507] -> w488 mode=indexing
            tunnel: w427 -> [w506]
            shift-right: [w504] -> w483
            shift-left: w496 -> [w503]
            i -> [w505]
            n130 = Pick Line(multi-line string=w506, line index=w505) -> (output string=w508:string)  [unwired: 1 in]
            n131 = call "Numeric String to Bytes.vi"("Type"=T3."U8", "String"=w508) -> ("error out"=w507:errorcluster, "Byte Data"=w502:u8[])  [unwired: 8 in]
            n132 = Build Array (concatenate)(w503, w502) -> (w504:u8[])
          }
          n133 = Pick Line(multi-line string=w427, line index=12) -> (output string=w485:string)  [unwired: 1 in]
          n134 = Pick Line(multi-line string=w427, line index=13) -> (output string=w479:string)  [unwired: 1 in]
          n135 = Pick Line(multi-line string=w427, line index=14) -> (output string=w474:string)  [unwired: 1 in]
          n136 = Pick Line(multi-line string=w427, line index=15) -> (output string=w471:string)  [unwired: 1 in]
          n137 = Pick Line(multi-line string=w427, line index=16) -> (output string=w468:string)  [unwired: 1 in]
          n138 = Pick Line(multi-line string=w427, line index=18) -> (output string=w457:string)  [unwired: 1 in]
          n139 = Bundle By Name(cluster=T4 {"fractional second"=0.0, "second"=0, "minute"=0, "hour"=0, "day of month"=0, "month"=0, "year"=0, "day of week"=0, "day of year"=0, "DST"=0} ("date time rec"), "month"=w453, "day of month"=w452, "year"=w451, "hour"=w447, "minute"=w449, "second"=w448, "day of week"=w445, "day of year"=w445, "DST"=w445, "fractional second"=w445) -> (w444:T4)
          n140 = Match Pattern(string=w485, regular expression="=") -> (after substring=w484:string)  [unwired: 1 in, 3 out]
          n141 = call "Numeric String to Bytes.vi"("Type"=T3."U16", "String"=w479) -> ("error out"=w477:errorcluster, "Byte Data"=w478:u8[])  [unwired: 8 in]
          n142 = call "Numeric String to Bytes.vi"("Type"=T3."U8", "String"=w474) -> ("error out"=w466:errorcluster, "Byte Data"=w463:u8[])  [unwired: 8 in]
          n143 = call "Numeric String to Bytes.vi"("Type"=T3."U8", "String"=w471) -> ("error out"=w465:errorcluster, "Byte Data"=w462:u8[])  [unwired: 8 in]
          n144 = call "Numeric String to Bytes.vi"("Type"=T3."U8", "String"=w468) -> ("error out"=w464:errorcluster, "Byte Data"=w461:u8[])  [unwired: 8 in]
          n145 = call "Numeric String to Bytes.vi"("Type"=T3."U8", "String"=w457) -> ("error out"=w431:errorcluster, "Byte Data"=w458:u8[])  [unwired: 8 in]
          n146 = call <vilib>:"Trim Whitespace.vi"("string"=w484) -> ("trimmed string"=w492:string)  [unwired: 1 in]
          n147 = String To Byte Array(string=w492) -> (unsigned byte array=w491:u8[])
          n148 = Date/Time To Seconds(2:w444) -> (0:w440:timestamp)  [unwired: 1 in]
          n149 = Replace Array Subset(array=w489, new element=w491, index=0) -> (w481:u8[])
          n150 = To Unsigned Quad Integer(1:w440) -> (0:w439:u64)
          n151 = Multiply(x=u64 1904 ("y"), y=u64 31556926) -> (x*y=w438:u64)
          n152 = Add(x=w439, y=w438) -> (x+y=w437:u64)
          n153 = Multiply(x=u64 10000000 ("y"), y=w437) -> (x*y=w435:u64)
          n154 = Number To Decimal String(number=w435) -> (decimal integer string=w432:string)  [unwired: 1 in]
          n155 = Concatenate Strings("MS_Date=" ("string"), w432) -> (w433:string)
          n156 = call "Numeric String to Bytes.vi"("Type"=T3."U64", "String"=w433) -> ("error out"=w430:errorcluster, "Byte Data"=w428:u8[])  [unwired: 8 in]
          n157 = Build Array (concatenate)(w483, w481, w478, w463, w462, w461, w423, w428, w458, w423) -> (w494:u8[])
          n158 = Build Array (concatenate)(w488, w477, w466, w465, w464, w443, w430, w431) -> (w487:errorcluster[])
          n159 = Merge Errors(w487) -> (w495:errorcluster)
        }
        frame "Get Pulse Constants" {
          # "Get Pulse Constants"
        }
        frame "Set Pulse Constants" {
          w513 = u8[] []  # DATA
          # "Set Pulse Constants"
          n160 = for {
            N: 11 -> [_]
            tunnel: w518 -> [w538]
            shift-right: [w534] -> w529
            shift-left: w513 -> [w535]
            tunnel: [w532] -> w516 mode=indexing
            i -> [w539]
            n161 = Pick Line(multi-line string=w538, line index=w539) -> (output string=w537:string)  [unwired: 1 in]
            n162 = call "Numeric String to Bytes.vi"("Type"=T3."U16", "String"=w537) -> ("error out"=w532:errorcluster, "Byte Data"=w533:u8[])  [unwired: 8 in]
            n163 = Build Array (concatenate)(w535, w533) -> (w534:u8[])
          }
          n164 = Pick Line(multi-line string=w518, line index=11) -> (output string=w526:string)  [unwired: 1 in]
          n165 = Pick Line(multi-line string=w518, line index=12) -> (output string=w523:string)  [unwired: 1 in]
          n166 = call "Numeric String to Bytes.vi"("Type"=T3."U8", "String"=w526) -> ("error out"=w514:errorcluster, "Byte Data"=w519:u8[])  [unwired: 8 in]
          n167 = call "Numeric String to Bytes.vi"("Type"=T3."U8", "String"=w523) -> ("error out"=w517:errorcluster, "Byte Data"=w520:u8[])  [unwired: 8 in]
          n168 = Build Array (concatenate)(w529, w519, w520) -> (w528:u8[])
          n169 = Build Array (concatenate)(w516, w514, w517) -> (w515:errorcluster[])
          n170 = Merge Errors(w515) -> (w527:errorcluster)
        }
        frame "Get Lead Limits" {
          # "Get Lead Limits"
        }
        frame "Set Lead Limits" {
          w543 = u8[] []  # DATA
          # "Set Lead Limits"
          n171 = for {
            N: 52 -> [_]
            tunnel: w546 -> [w556]
            shift-right: [w552] -> w544
            shift-left: w543 -> [w553]
            tunnel: [w550] -> w545 mode=indexing
            i -> [w557]
            n172 = Pick Line(multi-line string=w556, line index=w557) -> (output string=w555:string)  [unwired: 1 in]
            n173 = call "Numeric String to Bytes.vi"("Type"=T3."U16", "String"=w555) -> ("error out"=w550:errorcluster, "Byte Data"=w551:u8[])  [unwired: 8 in]
            n174 = Build Array (concatenate)(w553, w551) -> (w552:u8[])
          }
          n175 = Merge Errors(w545) -> (w547:errorcluster)
        }
        frame "Get Channel Calibrations" {
          # "Get Channel Calibrations"
          n176 = call "Numeric String to Bytes.vi"("Type"=T3."U8", "String"=w560) -> ("error out"=w561:errorcluster, "Byte Data"=w563:u8[])  [unwired: 8 in]
          n177 = Replace Array Subset(array=w559, new element=w563, index=0) -> (w558:u8[])
        }
        frame "Set Channel Calibrations" {
          w574 = u8[] []  # DATA
          # "Set Channel Calibrations"
          n178 = for {
            N: 52 -> [_]
            tunnel: w567 -> [w587]
            shift-right: [w583] -> w569
            shift-left: w574 -> [w584]
            tunnel: [w581] -> w575 mode=indexing
            i -> [w579]
            n179 = Increment(x=w579) -> (x+1=w580:i32)
            n180 = Pick Line(multi-line string=w587, line index=w580) -> (output string=w586:string)  [unwired: 1 in]
            n181 = call "Numeric String to Bytes.vi"("Type"=T3."U16", "String"=w586) -> ("error out"=w581:errorcluster, "Byte Data"=w582:u8[])  [unwired: 8 in]
            n182 = Build Array (concatenate)(w584, w582) -> (w583:u8[])
          }
          n183 = Pick Line(multi-line string=w567, line index=0) -> (output string=w573:string)  [unwired: 1 in]
          n184 = call "Numeric String to Bytes.vi"("Type"=T3."U16", "String"=w573) -> ("error out"=w566:errorcluster, "Byte Data"=w568:u8[])  [unwired: 8 in]
          n185 = Build Array (concatenate)(w568, w569) -> (w570:u8[])
          n186 = Merge Errors(w575, w566) -> (w576:errorcluster)
        }
        frame "Get Stim Asic HV Calibrations" {
          # "Get Stim ASIC HV Calibrations"
        }
        frame "Set Stim Asic HV Calibrations" {
          w591 = u8[] []  # DATA
          # "Set Stim ASIC HV Calibrations"
          n187 = for {
            N: 64 -> [_]
            tunnel: w594 -> [w604]
            shift-right: [w600] -> w592
            shift-left: w591 -> [w601]
            tunnel: [w598] -> w593 mode=indexing
            i -> [w605]
            n188 = Pick Line(multi-line string=w604, line index=w605) -> (output string=w603:string)  [unwired: 1 in]
            n189 = call "Numeric String to Bytes.vi"("Type"=T3."U16", "String"=w603) -> ("error out"=w598:errorcluster, "Byte Data"=w599:u8[])  [unwired: 8 in]
            n190 = Build Array (concatenate)(w601, w599) -> (w600:u8[])
          }
          n191 = Merge Errors(w593) -> (w595:errorcluster)
        }
        frame "Get CP Data" {
          # "Get CP Data"
          n192 = call "Numeric String to Bytes.vi"("Type"=T3."U8", "String"=w611) -> ("error out"=w610:errorcluster, "Byte Data"=w607:u8[])  [unwired: 8 in]
          n193 = Replace Array Subset(array=w612, new element=w607, index=0) -> (w609:u8[])
        }
        frame "Set CP Data" {
          # "Set CP Data"
          n194 = Array To Cluster(array=w616) -> (cluster=w614:T5)
          n195 = Pick Line(multi-line string=w620, line index=0) -> (output string=w622:string)  [unwired: 1 in]
          n196 = Cluster To Array(cluster=w614) -> (array=w615:u8[])
          n197 = call "Numeric String to Bytes.vi"("Type"=T3."U16", "String"=w622) -> ("error out"=w617:errorcluster, "Byte Data"=w618:u8[])  [unwired: 8 in]
          n198 = Build Array (concatenate)(w618, w615) -> (w619:u8[])
          n199 = Merge Errors(w617) -> (w624:errorcluster)
        }
        frame "Clear Log" {
          # "Clear Log"
          n200 = call "Numeric String to Bytes.vi"("Type"=T3."U8", "String"=w631) -> ("error out"=w630:errorcluster, "Byte Data"=w627:u8[])  [unwired: 8 in]
          n201 = Replace Array Subset(array=w632, new element=w627, index=0) -> (w629:u8[])
        }
        frame "Read Log" {
          # "Read Log"
          n202 = Pick Line(multi-line string=w635, line index=0) -> (output string=w645:string)  [unwired: 1 in]
          n203 = Pick Line(multi-line string=w635, line index=1) -> (output string=w642:string)  [unwired: 1 in]
          n204 = call "Numeric String to Bytes.vi"("Type"=T3."U16", "String"=w645) -> ("error out"=w639:errorcluster, "Byte Data"=w641:u8[])  [unwired: 8 in]
          n205 = call "Numeric String to Bytes.vi"("Type"=T3."U32", "String"=w642) -> ("error out"=w638:errorcluster, "Byte Data"=w634:u8[])  [unwired: 8 in]
          n206 = Build Array(w639, w638) -> (w637:errorcluster[])
          n207 = Build Array (concatenate)(w641, w634) -> (w640:u8[])
          n208 = Replace Array Subset(array=w650, new element=w640, index=0) -> (w649:u8[])
          n209 = Merge Errors(w637) -> (w636:errorcluster)
        }
        frame "Append Log" {
          # "Added a U8 Data"
          # "Changed to U16 from U8"
          # "Append Log"
          n210 = Pick Line(multi-line string=w654, line index=0) -> (output string=w683:string)  [unwired: 1 in]
          n211 = Pick Line(multi-line string=w654, line index=1) -> (output string=w680:string)  [unwired: 1 in]
          n212 = Pick Line(multi-line string=w654, line index=2) -> (output string=w670:string)  [unwired: 1 in]
          n213 = Pick Line(multi-line string=w654, line index=3) -> (output string=w667:string)  [unwired: 1 in]
          n214 = Pick Line(multi-line string=w654, line index=4) -> (output string=w664:string)  [unwired: 1 in]
          n215 = Pick Line(multi-line string=w654, line index=5) -> (output string=w657:string)  [unwired: 1 in]
          n216 = call "Numeric String to Bytes.vi"("Type"=T3."U16", "String"=w683) -> ("error out"=w676:errorcluster, "Byte Data"=w679:u8[])  [unwired: 8 in]
          n217 = call "Numeric String to Bytes.vi"("Type"=T3."U16", "String"=w680) -> ("error out"=w675:errorcluster, "Byte Data"=w677:u8[])  [unwired: 8 in]
          n218 = call "Numeric String to Bytes.vi"("Type"=T3."U8", "String"=w670) -> ("error out"=w660:errorcluster, "Byte Data"=w661:u8[])  [unwired: 8 in]
          n219 = call "Numeric String to Bytes.vi"("Type"=T3."U8", "String"=w667) -> ("error out"=w659:errorcluster, "Byte Data"=w662:u8[])  [unwired: 8 in]
          n220 = call "Numeric String to Bytes.vi"("Type"=T3."U8", "String"=w664) -> ("error out"=w658:errorcluster, "Byte Data"=w663:u8[])  [unwired: 8 in]
          n221 = call "Numeric String to Bytes.vi"("Type"=T3."U8", "String"=w657) -> ("error out"=w653:errorcluster, "Byte Data"=w652:u8[])  [unwired: 8 in]
          n222 = Build Array (concatenate)(w679, w677, w661, w662, w663, w652) -> (w678:u8[])
          n223 = Build Array(w676, w675, w660, w659, w658, w653) -> (w674:errorcluster[])
          n224 = Replace Array Subset(array=w688, new element=w678, index=0) -> (w687:u8[])
          n225 = Merge Errors(w674) -> (w673:errorcluster)
        }
        frame "Get Patient Program Runtime" {
          # "Get Patient Program Run-Time"
          n226 = call "Numeric String to Bytes.vi"("Type"=T3."U8", "String"=w695) -> ("error out"=w694:errorcluster, "Byte Data"=w691:u8[])  [unwired: 8 in]
          n227 = Replace Array Subset(array=w696, new element=w691, index=0) -> (w693:u8[])
        }
        frame "Set Patient Program Runtime" {
          # "Set Patient Program Run-Time"
          n228 = Pick Line(multi-line string=w698, line index=0) -> (output string=w709:string)  [unwired: 1 in]
          n229 = Pick Line(multi-line string=w698, line index=1) -> (output string=w706:string)  [unwired: 1 in]
          n230 = call "Numeric String to Bytes.vi"("Type"=T3."U16", "String"=w709) -> ("error out"=w702:errorcluster, "Byte Data"=w705:u8[])  [unwired: 8 in]
          n231 = call "Numeric String to Bytes.vi"("Type"=T3."U32", "String"=w706) -> ("error out"=w701:errorcluster, "Byte Data"=w703:u8[])  [unwired: 8 in]
          n232 = Build Array (concatenate)(w705, w703) -> (w704:u8[])
          n233 = Build Array(w702, w701) -> (w700:errorcluster[])
          n234 = Replace Array Subset(array=w714, new element=w704, index=0) -> (w713:u8[])
          n235 = Merge Errors(w700) -> (w699:errorcluster)
        }
        frame "Impedance Measurement" {
          # "Changed to U16 from U8"
          # "Impedance Measurement"
          n236 = Pick Line(multi-line string=w716, line index=0) -> (output string=w732:string)  [unwired: 1 in]
          n237 = Pick Line(multi-line string=w716, line index=1) -> (output string=w729:string)  [unwired: 1 in]
          n238 = Pick Line(multi-line string=w716, line index=2) -> (output string=w719:string)  [unwired: 1 in]
          n239 = call "Numeric String to Bytes.vi"("Type"=T3."U8", "String"=w732) -> ("error out"=w725:errorcluster, "Byte Data"=w728:u8[])  [unwired: 8 in]
          n240 = call "Numeric String to Bytes.vi"("Type"=T3."U8", "String"=w729) -> ("error out"=w724:errorcluster, "Byte Data"=w726:u8[])  [unwired: 8 in]
          n241 = call "Numeric String to Bytes.vi"("Type"=T3."U8", "String"=w719) -> ("error out"=w717:errorcluster, "Byte Data"=w718:u8[])  [unwired: 8 in]
          n242 = Build Array (concatenate)(w728, w726, w718) -> (w727:u8[])
          n243 = Replace Array Subset(array=w737, new element=w727, index=0) -> (w736:u8[])
          n244 = Build Array(w725, w724, w717) -> (w723:errorcluster[])
          n245 = Merge Errors(w723) -> (w722:errorcluster)
        }
        frame "Enter Storage Mode" {
          # "Enter Storage Mode"
        }
        frame "Echo Short" {
          # "Echo Short"
          n246 = Array Subset(array=w746, index=0, length=8) -> (w743:u8[])
        }
        frame "Echo Long" {
          # "Echo Long"
          n247 = Array Subset(array=w752, index=0, length=256) -> (w749:u8[])
        }
        frame "Get General Calibration" {
          # "Get General Calibration"
        }
        frame "Set General Calibration" {
          w757 = u8[] []  # DATA
          # "Set General Calibration"
          n248 = disable-structure shown="Enabled" {
            disable-tunnel: [w794 w846] -> w761
            disable-tunnel: [w790 w845] -> w759
            disable-tunnel: w758 -> [w777 w848]
            disable-tunnel: w757 -> [w763 w847]
            frame Disabled {
              n249 = for {
                N: 15 -> [_]
                tunnel: [w841] -> w795 mode=indexing
                tunnel: w777 -> [w840]
                shift-right: [w837] -> w789
                shift-left: w763 -> [w838]
                tunnel: [w836] -> w773
                i -> [w836]
                n250 = Pick Line(multi-line string=w840, line index=w836) -> (output string=w842:string)  [unwired: 1 in]
                n251 = call "Numeric String to Bytes.vi"("Type"=T3."U16", "String"=w842) -> ("error out"=w841:errorcluster, "Byte Data"=w839:u8[])  [unwired: 8 in]
                n252 = Build Array (concatenate)(w838, w839) -> (w837:u8[])
              }
              n253 = Increment(x=w773) -> (x+1=w772:i32)
              n254 = for {
                N: 12 -> [_]
                tunnel: [w803] -> w775 mode=indexing
                tunnel: w777 -> [w802]
                shift-right: [w799] -> w774
                shift-left: w763 -> [w800]
                tunnel: w772 -> [w797]
                tunnel: [w796] -> w770
                i -> [w796]
                n255 = Add(x=w797, y=w796) -> (x+y=w798:i32)
                n256 = Pick Line(multi-line string=w802, line index=w798) -> (output string=w804:string)  [unwired: 1 in]
                n257 = call "Numeric String to Bytes.vi"("Type"=T3."U16", "String"=w804) -> ("error out"=w803:errorcluster, "Byte Data"=w801:u8[])  [unwired: 8 in]
                n258 = Build Array (concatenate)(w800, w801) -> (w799:u8[])
              }
              n259 = Increment(x=w770) -> (x+1=w771:i32)
              n260 = for {
                N: 15 -> [_]
                tunnel: [w833] -> w787 mode=indexing
                tunnel: w777 -> [w832]
                shift-right: [w829] -> w788
                shift-left: w763 -> [w830]
                tunnel: w771 -> [w827]
                tunnel: [w826] -> w769
                i -> [w826]
                n261 = Add(x=w827, y=w826) -> (x+y=w828:i32)
                n262 = Pick Line(multi-line string=w832, line index=w828) -> (output string=w834:string)  [unwired: 1 in]
                n263 = call "Numeric String to Bytes.vi"("Type"=T3."U16", "String"=w834) -> ("error out"=w833:errorcluster, "Byte Data"=w831:u8[])  [unwired: 8 in]
                n264 = Build Array (concatenate)(w830, w831) -> (w829:u8[])
              }
              n265 = Increment(x=w769) -> (x+1=w768:i32)
              n266 = for {
                N: 5 -> [_]
                tunnel: [w823] -> w784 mode=indexing
                tunnel: w777 -> [w822]
                shift-right: [w819] -> w785
                shift-left: w763 -> [w820]
                tunnel: w768 -> [w817]
                tunnel: [w816] -> w766
                i -> [w816]
                n267 = Add(x=w817, y=w816) -> (x+y=w818:i32)
                n268 = Pick Line(multi-line string=w822, line index=w818) -> (output string=w824:string)  [unwired: 1 in]
                n269 = call "Numeric String to Bytes.vi"("Type"=T3."U16", "String"=w824) -> ("error out"=w823:errorcluster, "Byte Data"=w821:u8[])  [unwired: 8 in]
                n270 = Build Array (concatenate)(w820, w821) -> (w819:u8[])
              }
              n271 = Increment(x=w766) -> (x+1=w767:i32)
              n272 = for {
                N: 5 -> [_]
                tunnel: [w813] -> w781 mode=indexing
                tunnel: w777 -> [w812]
                shift-right: [w809] -> w782
                shift-left: _ -> [w810]
                tunnel: w767 -> [w807]
                tunnel: [w806] -> w765
                i -> [w806]
                n273 = Add(x=w807, y=w806) -> (x+y=w808:i32)
                n274 = Pick Line(multi-line string=w812, line index=w808) -> (output string=w814:string)  [unwired: 1 in]
                n275 = call "Numeric String to Bytes.vi"("Type"=T3."U16", "String"=w814) -> ("error out"=w813:errorcluster, "Byte Data"=w811:u8[])  [unwired: 8 in]
                n276 = Build Array (concatenate)(w810, w811) -> (w809:u8[])
              }
              n277 = Increment(x=w765) -> (x+1=w764:i32)
              n278 = Pick Line(multi-line string=w777, line index=w764) -> (output string=w792:string)  [unwired: 1 in]
              n279 = call "Numeric String to Bytes.vi"("Type"=T3."U16", "String"=w792) -> ("error out"=w780:errorcluster, "Byte Data"=w779:u8[])  [unwired: 8 in]
              n280 = Build Array (concatenate)(w789, w774, w788, w785, w782, w779) -> (w790:u8[])
              n281 = Build Array (concatenate)(w795, w775, w787, w784, w781, w780) -> (w794:errorcluster[])
            }
            frame Enabled {
              n282 = for {
                N: 55 -> [_]
                tunnel: [w854] -> w846 mode=indexing
                tunnel: w848 -> [w853]
                shift-right: [w850] -> w845
                shift-left: w847 -> [w851]
                i -> [w849]
                n283 = Pick Line(multi-line string=w853, line index=w849) -> (output string=w855:string)  [unwired: 1 in]
                n284 = call "Numeric String to Bytes.vi"("Type"=T3."U16", "String"=w855) -> ("error out"=w854:errorcluster, "Byte Data"=w852:u8[])  [unwired: 8 in]
                n285 = Build Array (concatenate)(w851, w852) -> (w850:u8[])
              }
            }
          }
          n286 = Merge Errors(w761) -> (w760:errorcluster)
        }
        frame "Get Trim List" {
          # "Changed to U8 from U16"
          # "Get Trim List"
          n287 = call "Numeric String to Bytes.vi"("Type"=T3."U8", "String"=w859) -> ("error out"=w858:errorcluster, "Byte Data"=w862:u8[])  [unwired: 8 in]
          n288 = Replace Array Subset(array=w860, new element=w862, index=0) -> (w857:u8[])
        }
        frame "Set Trim List" {
          w887 = u8[] []  # DATA
          # "Set Trim List"
          n289 = Pick Line(multi-line string=w868, line index=0) -> (output string=w886:string)  [unwired: 1 in]
          n290 = Pick Line(multi-line string=w868, line index=1) -> (output string=w884:string)  [unwired: 1 in]
          n291 = call "Numeric String to Bytes.vi"("Type"=T3."U8", "String"=w886) -> ("error out"=w874:errorcluster, "Byte Data"=w870:u8[])  [unwired: 8 in]
          n292 = call "Numeric String to Bytes.vi"("Type"=T3."U8", "String"=w884) -> ("error out"=w873:errorcluster, "Byte Data"=w882:u8[])  [unwired: 8 in]
          n293 = Index Array(array=w870, index=0) -> (element=w869:u8)
          n294 = Index Array(array=w882, index=0) -> (element=w881:u8)
          n295 = case shown="0, Default" w869 {
            tunnel: w887 -> [w900 w928]
            tunnel: w881 -> [w888 w918]
            tunnel: w868 -> [w899 w927]
            tunnel: [w898 w926] -> w877
            tunnel: [w897 w926] -> w875
            tunnel: [w893 w924] -> w872
            frame 0, Default {
              # "\"Normal\" Trim List, with Address:Data tuples"
              n296 = for {
                N: w888 -> [_]
                tunnel: w899 -> [w901]
                shift-right: [w914] -> w894
                shift-left: w900 -> [w915]
                tunnel: [w912] -> w898 mode=indexing
                tunnel: [w909] -> w897 mode=indexing
                i -> [w903]
                w904 = 2 ("y")
                n297 = Multiply(x=w904, y=w903) -> (x*y=w905:i32)
                n298 = Add(x=w904, y=w905) -> (x+y=w908:i32)
                n299 = Add(x=w905, y=3) -> (x+y=w907:i32)
                n300 = Pick Line(multi-line string=w901, line index=w908) -> (output string=w917:string)  [unwired: 1 in]
                n301 = Pick Line(multi-line string=w901, line index=w907) -> (output string=w911:string)  [unwired: 1 in]
                n302 = call "Numeric String to Bytes.vi"("Type"=T3."U16", "String"=w917) -> ("error out"=w912:errorcluster, "Byte Data"=w913:u8[])  [unwired: 8 in]
                n303 = call "Numeric String to Bytes.vi"("Type"=T3."U8", "String"=w911) -> ("error out"=w909:errorcluster, "Byte Data"=w902:u8[])  [unwired: 8 in]
                n304 = Build Array (concatenate)(w915, w913, w902) -> (w914:u8[])
              }
              n305 = Multiply(x=u8 3, y=w888) -> (x*y=w890:u8)
              n306 = Subtract(x=u8 96, y=w890) -> (x-y=w895:u8)
              n307 = Initialize Array(u8 0, w895) -> (w892:u8[])
              n308 = Build Array (concatenate)(w894, w892) -> (w893:u8[])
            }
            frame 2 {
              n309 = Decrement(x=w918) -> (x-1=w925:u8)
              n310 = for {
                N: w925 -> [_]
                tunnel: w927 -> [w932]
                shift-right: [w937] -> w923
                shift-left: w928 -> [w938]
                tunnel: [w935] -> w926 mode=indexing
                i -> [w931]
                # "\"Stim Trims\" List - Five U8's and a U16"
                n311 = Add(x=2 ("y"), y=w931) -> (x+y=w934:i32)
                n312 = Equal?(x=w931, y=5) -> (x = y?=w929:bool)
                n313 = Pick Line(multi-line string=w932, line index=w934) -> (output string=w939:string)  [unwired: 1 in]
                n314 = case shown="True" w929 {
                  tunnel: w939 -> [w942 w948]
                  tunnel: [w941 w944] -> w936
                  tunnel: [w940 w946] -> w935
                  frame False {
                    # "U8 Stim Trim"
                    n315 = call "Numeric String to Bytes.vi"("Type"=T3."U8", "String"=w942) -> ("error out"=w940:errorcluster, "Byte Data"=w941:u8[])  [unwired: 8 in]
                  }
                  frame True {
                    # "U16 Gain Trim"
                    n316 = call "Numeric String to Bytes.vi"("Type"=T3."U16", "String"=w948) -> ("error out"=w946:errorcluster, "Byte Data"=w945:u8[])  [unwired: 8 in]
                    n317 = Reverse 1D Array(array=w945) -> (reversed array=w944:u8[])
                  }
                }
                n318 = Build Array (concatenate)(w938, w936) -> (w937:u8[])
              }
              n319 = Subtract(x=96, y=w918) -> (x-y=w919:i32)
              n320 = Initialize Array(u8 0, w919) -> (w921:u8[])
              n321 = Build Array (concatenate)(w923, w921) -> (w924:u8[])
            }
          }
          n322 = Build Array (concatenate)(w870, w882, w872) -> (w867:u8[])
          n323 = Build Array (concatenate)(w877, w875, w874, w873) -> (w876:errorcluster[])
          n324 = Merge Errors(w876) -> (w865:errorcluster)
        }
        frame "Get Counter" {
          # "Get Counter"
          n325 = call "Numeric String to Bytes.vi"("Type"=T3."U8", "String"=w954) -> ("error out"=w953:errorcluster, "Byte Data"=w950:u8[])  [unwired: 8 in]
          n326 = Replace Array Subset(array=w955, new element=w950, index=0) -> (w952:u8[])
        }
        frame "Set Counter" {
          # "Set Counter"
          n327 = Pick Line(multi-line string=w959, line index=0) -> (output string=w969:string)  [unwired: 1 in]
          n328 = Pick Line(multi-line string=w959, line index=1) -> (output string=w966:string)  [unwired: 1 in]
          n329 = call "Numeric String to Bytes.vi"("Type"=T3."U8", "String"=w969) -> ("error out"=w963:errorcluster, "Byte Data"=w958:u8[])  [unwired: 8 in]
          n330 = call "Numeric String to Bytes.vi"("Type"=T3."U32", "String"=w966) -> ("error out"=w962:errorcluster, "Byte Data"=w964:u8[])  [unwired: 8 in]
          n331 = Build Array (concatenate)(w958, u8[] [0] ("array"), w964) -> (w965:u8[])
          n332 = Build Array(w963, w962) -> (w961:errorcluster[])
          n333 = Replace Array Subset(array=w974, new element=w965, index=0) -> (w973:u8[])
          n334 = Merge Errors(w961) -> (w960:errorcluster)
        }
        frame "Get Test Stimulation" {
          # "Get Test Stimulation"
        }
        frame "Set Test Stimulation" {
          w996 = u8[] []  # DATA
          # "Set Test Stimulation"
          n335 = for {
            N: 4 -> [_]
            shift-right: [w1042] -> w980
            shift-left: w996 -> [w1044]
            tunnel: w984 -> [w1021]
            shift-right: [w1017] -> _
            shift-left: 3 ("line index") -> [w1047]
            tunnel: [w1039] -> w1001 mode=indexing
            w1040 = u8[] []  # DATA
            n336 = Increment(x=w1047) -> (x+1=w1038:i32)
            n337 = Pick Line(multi-line string=w1021, line index=w1047) -> (output string=w1045:string)  [unwired: 1 in]
            n338 = for {
              N: 26 -> [_]
              tunnel: w1021 -> [w1056]
              shift-right: [w1051] -> w1019
              shift-left: w1040 -> [w1052]
              shift-right: [w1049] -> w1029
              shift-left: w1038 -> [w1050]
              tunnel: [w1048] -> _ mode=indexing
              n339 = Pick Line(multi-line string=w1056, line index=w1050) -> (output string=w1054:string)  [unwired: 1 in]
              n340 = Increment(x=w1050) -> (x+1=w1049:i32)
              n341 = call "Numeric String to Bytes.vi"("Type"=T3."I8", "String"=w1054) -> ("error out"=w1048:errorcluster, "Byte Data"=w1053:u8[])  [unwired: 8 in]
              n342 = Build Array (concatenate)(w1052, w1053) -> (w1051:u8[])
            }
            n343 = Increment(x=w1029) -> (x+1=w1028:i32)
            n344 = Pick Line(multi-line string=w1021, line index=w1029) -> (output string=w1037:string)  [unwired: 1 in]
            n345 = Increment(x=w1028) -> (x+1=w1027:i32)
            n346 = Pick Line(multi-line string=w1021, line index=w1028) -> (output string=w1034:string)  [unwired: 1 in]
            n347 = Increment(x=w1027) -> (x+1=w1025:i32)
            n348 = Pick Line(multi-line string=w1021, line index=w1027) -> (output string=w1032:string)  [unwired: 1 in]
            n349 = Increment(x=w1025) -> (x+1=w1020:i32)
            n350 = Pick Line(multi-line string=w1021, line index=w1025) -> (output string=w1031:string)  [unwired: 1 in]
            n351 = call "Numeric String to Bytes.vi"("Type"=T3."U16", "String"=w1045) -> ("error out"=w1010:errorcluster, "Byte Data"=w1043:u8[])  [unwired: 8 in]
            n352 = Increment(x=w1020) -> (x+1=w1018:i32)
            n353 = Pick Line(multi-line string=w1021, line index=w1020) -> (output string=w1030:string)  [unwired: 1 in]
            n354 = Pick Line(multi-line string=w1021, line index=w1018) -> (output string=w1022:string)  [unwired: 1 in]
            n355 = call "Numeric String to Bytes.vi"("Type"=T3."U16", "String"=w1037) -> ("error out"=w1009:errorcluster, "Byte Data"=w1016:u8[])  [unwired: 8 in]
            n356 = call "Numeric String to Bytes.vi"("Type"=T3."U8", "String"=w1034) -> ("error out"=w1008:errorcluster, "Byte Data"=w1015:u8[])  [unwired: 8 in]
            n357 = call "Numeric String to Bytes.vi"("Type"=T3."U8", "String"=w1032) -> ("error out"=w1007:errorcluster, "Byte Data"=w1014:u8[])  [unwired: 8 in]
            n358 = call "Numeric String to Bytes.vi"("Type"=T3."U16", "String"=w1031) -> ("error out"=w1006:errorcluster, "Byte Data"=w1013:u8[])  [unwired: 8 in]
            n359 = call "Numeric String to Bytes.vi"("Type"=T3."U16", "String"=w1030) -> ("error out"=w1005:errorcluster, "Byte Data"=w1012:u8[])  [unwired: 8 in]
            n360 = call "Numeric String to Bytes.vi"("Type"=T3."U8", "String"=w1022) -> ("error out"=w1004:errorcluster, "Byte Data"=w1011:u8[])  [unwired: 8 in]
            n361 = Build Array (concatenate)(w1044, w1043, w1019, w1016, w1015, w1014, w1013, w1012, w1011, u8[] [0] ("array")) -> (w1042:u8[])
            n362 = Merge Errors(w1010, w1009, w1008, w1007, w1006, w1005, w1004) -> (w1039:errorcluster)
            n363 = Increment(x=w1018) -> (x+1=w1017:i32)
          }
          n364 = Pick Line(multi-line string=w984, line index=2) -> (output string=w985:string)  [unwired: 1 in]
          n365 = Pick Line(multi-line string=w984, line index=0) -> (output string=w991:string)  [unwired: 1 in]
          n366 = Pick Line(multi-line string=w984, line index=1) -> (output string=w994:string)  [unwired: 1 in]
          n367 = call "Numeric String to Bytes.vi"("Type"=T3."U8", "String"=w985) -> ("Byte Data"=w983:u8[])  [unwired: 8 in, 1 out]
          n368 = call "Numeric String to Bytes.vi"("Type"=T3."U8", "String"=w991) -> ("error out"=w999:errorcluster, "Byte Data"=w988:u8[])  [unwired: 8 in]
          n369 = call "Numeric String to Bytes.vi"("Type"=T3."U8", "String"=w994) -> ("error out"=w1000:errorcluster, "Byte Data"=w998:u8[])  [unwired: 8 in]
          n370 = Build Array (concatenate)(w988, w998, w983, u8[] [0] ("array"), w980) -> (w981:u8[])
          n371 = Merge Errors(w999, w1000, w1001) -> (w982:errorcluster)
        }
        frame "Get Titration Stimulation" {
          # "Get Titration Stimulation"
        }
        frame "Set Titration Stimulation" {
          w1070 = u8[] []  # DATA
          # "Set Titration Stimulation"
          n372 = for {
            N: 4 -> [_]
            shift-right: [w1090] -> w1065
            shift-left: w1070 -> [w1093]
            tunnel: w1069 -> [w1079]
            shift-right: [w1084] -> _
            shift-left: 2 ("line index") -> [w1098]
            tunnel: [w1080] -> w1061 mode=indexing
            w1086 = u8[] []  # DATA
            n373 = Increment(x=w1098) -> (x+1=w1088:i32)
            n374 = Pick Line(multi-line string=w1079, line index=w1098) -> (output string=w1095:string)  [unwired: 1 in]
            n375 = Pick Line(multi-line string=w1079, line index=w1088) -> (output string=w1094:string)  [unwired: 1 in]
            n376 = Increment(x=w1088) -> (x+1=w1087:i32)
            n377 = call "Numeric String to Bytes.vi"("Type"=T3."U16", "String"=w1095) -> ("error out"=w1083:errorcluster, "Byte Data"=w1092:u8[])  [unwired: 8 in]
            n378 = call "Numeric String to Bytes.vi"("Type"=T3."U16", "String"=w1094) -> ("error out"=w1082:errorcluster, "Byte Data"=w1091:u8[])  [unwired: 8 in]
            n379 = for {
              N: 26 -> [_]
              tunnel: w1079 -> [w1107]
              shift-right: [w1102] -> w1085
              shift-left: w1086 -> [w1103]
              shift-right: [w1100] -> w1084
              shift-left: w1087 -> [w1101]
              tunnel: [w1099] -> w1081 mode=indexing
              n380 = Pick Line(multi-line string=w1107, line index=w1101) -> (output string=w1105:string)  [unwired: 1 in]
              n381 = Increment(x=w1101) -> (x+1=w1100:i32)
              n382 = call "Numeric String to Bytes.vi"("Type"=T3."I8", "String"=w1105) -> ("error out"=w1099:errorcluster, "Byte Data"=w1104:u8[])  [unwired: 8 in]
              n383 = Build Array (concatenate)(w1103, w1104) -> (w1102:u8[])
            }
            n384 = Build Array (concatenate)(w1093, w1092, w1091, w1085) -> (w1090:u8[])
            n385 = Merge Errors(w1083, w1082, w1081) -> (w1080:errorcluster)
          }
          n386 = Pick Line(multi-line string=w1069, line index=0) -> (output string=w1075:string)  [unwired: 1 in]
          n387 = Pick Line(multi-line string=w1069, line index=1) -> (output string=w1072:string)  [unwired: 1 in]
          n388 = call "Numeric String to Bytes.vi"("Type"=T3."U8", "String"=w1075) -> ("error out"=w1063:errorcluster, "Byte Data"=w1067:u8[])  [unwired: 8 in]
          n389 = call "Numeric String to Bytes.vi"("Type"=T3."U8", "String"=w1072) -> ("error out"=w1062:errorcluster, "Byte Data"=w1066:u8[])  [unwired: 8 in]
          n390 = Build Array (concatenate)(w1067, w1066, w1065) -> (w1064:u8[])
          n391 = Merge Errors(w1063, w1062, w1061) -> (w1060:errorcluster)
        }
        frame "Get Ramp Time" {
          # "Get Ramp Time"
        }
        frame "Set Ramp Time" {
          # "Set Ramp Time"
          n392 = call "Numeric String to Bytes.vi"("Type"=T3."U16", "String"=w1115) -> ("error out"=w1111:errorcluster, "Byte Data"=w1113:u8[])  [unwired: 8 in]
          n393 = Replace Array Subset(array=w1114, new element=w1113, index=0) -> (w1112:u8[])
        }
        frame "Get VBAT" {
          # "Get VBAT"
        }
        frame "Set Software Description Block" {
          # "Set Software Description Block"
        }
        frame "Get Software Description Block" {
          # "Get Software Description Block"
        }
        frame "Write Memory" {
          # "Write Memory"
          n394 = Pick Line(multi-line string=w1143, line index=0) -> (output string=w1150:string)  [unwired: 1 in]
          n395 = Pick Line(multi-line string=w1143, line index=1) -> (output string=w1147:string)  [unwired: 1 in]
          n396 = call "Numeric String to Bytes.vi"("Type"=T3."U32", "String"=w1150) -> ("error out"=w1145:errorcluster, "Byte Data"=w1146:u8[])  [unwired: 8 in]
          n397 = call "Numeric String to Bytes.vi"("Type"=T3."U16", "String"=w1147) -> ("error out"=w1144:errorcluster, "Byte Data"=w1138:u8[])  [unwired: 8 in]
          n398 = Merge Errors(w1145, w1144) -> (w1142:errorcluster)
          n399 = Array To Cluster(array=w1138) -> (cluster=w1137:T6)
          n400 = Unbundle By Name(w1137) -> ("Byte Data[1]"=w1136:u8, "Byte Data[0]"=w1135:u8)
          n401 = Join Numbers(hi=w1136, lo=w1135) -> ((hi.lo)=w1134:u16)
          n402 = Array Subset(array=w1139, index=0, length=w1134) -> (w1140:u8[])
          n403 = Build Array (concatenate)(w1146, w1138, w1140) -> (w1132:u8[])
          n404 = Array Size(array=w1131) -> (size(s)=w1130:i32)
          n405 = Array Size(array=w1132) -> (size(s)=w1129:i32)
          n406 = Greater?(x=w1130, y=w1129) -> (0:w1128:bool)
          n407 = case shown="False" w1128 {
            tunnel: [w1154 w1157] -> w1133
            tunnel: w1132 -> [w1154 w1156]
            tunnel: w1131 -> [_ w1155]
            frame False {
            }
            frame True {
              n408 = Replace Array Subset(array=w1155, new element=w1156, index=0) -> (w1157:u8[])
            }
          }
        }
        frame "Read Memory" {
          # "Read Memory"
          n409 = Pick Line(multi-line string=w1170, line index=0) -> (output string=w1172:string)  [unwired: 1 in]
          n410 = Pick Line(multi-line string=w1170, line index=1) -> (output string=w1168:string)  [unwired: 1 in]
          n411 = call "Numeric String to Bytes.vi"("Type"=T3."U32", "String"=w1172) -> ("error out"=w1163:errorcluster, "Byte Data"=w1165:u8[])  [unwired: 8 in]
          n412 = call "Numeric String to Bytes.vi"("Type"=T3."U16", "String"=w1168) -> ("error out"=w1162:errorcluster, "Byte Data"=w1164:u8[])  [unwired: 8 in]
          n413 = Build Array (concatenate)(w1165, w1164) -> (w1166:u8[])
          n414 = Merge Errors(w1163, w1162) -> (w1161:errorcluster)
          n415 = Replace Array Subset(array=w1160, new element=w1166, index=0) -> (w1159:u8[])
        }
        frame "Reset xPG" {
          # "Reset xPG"
        }
        frame "Erase Flash Block" {
          # "Erase Flash Block"
        }
        frame "Write Vectors" {
          # "Write Vectors"
        }
        frame "Read Vectors" {
          # "Read Vectors"
        }
        frame "Diagnostic Data" {
          # "Diagnostic  Data"
          n416 = Pick Line(multi-line string=w1200, line index=0) -> (output string=w1201:string)  [unwired: 1 in]
          n417 = Pick Line(multi-line string=w1200, line index=1) -> (output string=w1197:string)  [unwired: 1 in]
          n418 = call "Numeric String to Bytes.vi"("Type"=T3."U8", "String"=w1201) -> ("error out"=w1194:errorcluster, "Byte Data"=w1196:u8[])  [unwired: 8 in]
          n419 = call "Numeric String to Bytes.vi"("Type"=T3."U8", "String"=w1197) -> ("error out"=w1193:errorcluster, "Byte Data"=w1195:u8[])  [unwired: 8 in]
          n420 = Build Array (concatenate)(w1196, w1195) -> (w1189:u8[])
          n421 = Merge Errors(w1194, w1193) -> (w1192:errorcluster)
          n422 = Replace Array Subset(array=w1191, new element=w1189, index=0) -> (w1188:u8[])
        }
        frame "Set Background Impedance" {
          # "Set Background Impedance"
          n423 = Pick Line(multi-line string=w1208, line index=0) -> (output string=w1211:string)  [unwired: 1 in]
          n424 = Pick Line(multi-line string=w1208, line index=1) -> (output string=w1209:string)  [unwired: 1 in]
          n425 = call "Numeric String to Bytes.vi"("Type"=T3."U8", "String"=w1211) -> ("error out"=w1207:errorcluster, "Byte Data"=w1216:u8[])  [unwired: 8 in]
          n426 = call "Numeric String to Bytes.vi"("Type"=T3."U8", "String"=w1209) -> ("error out"=w1206:errorcluster, "Byte Data"=w1214:u8[])  [unwired: 8 in]
          n427 = Build Array (concatenate)(w1216, w1214) -> (w1213:u8[])
          n428 = Merge Errors(w1207, w1206) -> (w1205:errorcluster)
        }
        frame "Inject Event" {
          # "Inject Event"
          n429 = Pick Line(multi-line string=w1222, line index=0) -> (output string=w1225:string)  [unwired: 1 in]
          n430 = Pick Line(multi-line string=w1222, line index=1) -> (output string=w1223:string)  [unwired: 1 in]
          n431 = call "Numeric String to Bytes.vi"("Type"=T3."U16", "String"=w1225) -> ("error out"=w1221:errorcluster, "Byte Data"=w1230:u8[])  [unwired: 8 in]
          n432 = call "Numeric String to Bytes.vi"("Type"=T3."U16", "String"=w1223) -> ("error out"=w1220:errorcluster, "Byte Data"=w1228:u8[])  [unwired: 8 in]
          n433 = Build Array (concatenate)(w1230, w1228) -> (w1227:u8[])
          n434 = Merge Errors(w1221, w1220) -> (w1219:errorcluster)
        }
        frame "Get Background Impedence " {
          # "Get Background Impedance"
        }
        frame "Set Test Waveform" {
        }
        frame "Calibrate Channel" {
        }
        frame "Get Log Range" {
          n435 = Pick Line(multi-line string=w1244, line index=0) -> (output string=w1247:string)  [unwired: 1 in]
          n436 = call "Numeric String to Bytes.vi"("Type"=T3."U8", "String"=w1247) -> ("error out"=w1242:errorcluster, "Byte Data"=w1243:u8[])  [unwired: 8 in]
          n437 = Replace Array Subset(array=w1246, new element=w1243, index=0) -> (w1245:u8[])
        }
        frame "Reserved 0x55" {
        }
        frame "Reserved 0x56" {
        }
        frame "MICS Options" {
        }
        frame "Pair PPC" {
        }
        frame "Pair POP" {
        }
        frame "Stop Bootloader" {
        }
        frame "Tune MICS" {
        }
        frame "MICS Diagnostics" {
        }
        frame "Undefined" {
        }
        frame "<reserved 2>" {
        }
        frame "<reserved 3>" {
        }
        frame "<reserved 4>" {
        }
        frame "<reserved 5>" {
        }
        frame "<reserved 6>" {
        }
        frame "<reserved 7>" {
        }
        frame "<reserved 8>" {
        }
        frame "<reserved 9>" {
        }
      }
      n438 = Increment(x=w15) -> (x+1=w3:T1)
      n439 = while {
        tunnel: w3 -> [w20]
        tunnel: "EXID" -> [w19]
        shift-right: [w21] -> _
        shift-left: w13 -> [w22]
        tunnel: w10 -> [w17]
        tunnel: [w16] -> w12 mode=indexing
        i -> [w23]
        stop <- w18 continue-if-true
        n440 = case shown="1, Default" w23 {
          tunnel: w22 -> [w46 w56]
          tunnel: [w45 w60] -> w21
          tunnel: w20 -> [w26 _]
          tunnel: w19 -> [w42 _]
          tunnel: [w43 w58] -> w18
          tunnel: w17 -> [w38 w50]
          tunnel: [w29 w52] -> w16
          frame 0 {
            n441 = Split Number(x=w42) -> (hi(x)=w41:u16, lo(x)=w40:u16)
            n442 = Array To Cluster(array=w38) -> (cluster=w39:T7)
            n443 = Split Number(x=w41) -> (lo(x)=w36:u8)  [unwired: 1 out]
            n444 = Split Number(x=w40) -> (hi(x)=w37:u8, lo(x)=w35:u8)
            n445 = Delete From Array(array=w46, length=8, index=0) -> (deleted portion=w31:u8[], array with subset deleted=w45:u8[])
            n446 = Split Number(x=w26) -> (hi(x)=w27:u8, lo(x)=w28:u8)
            n447 = Bundle By Name(cluster=w39, "DATA[5]"=w27, "DATA[4]"=w28, "DATA[3]"=w36, "DATA[2]"=w37, "DATA[1]"=w35, "DATA[0]"=1) -> (w33:T7)
            n448 = Cluster To Array(cluster=w33) -> (array=w30:u8[])
            n449 = Array Size(array=w45) -> (size(s)=w44:i32)
            n450 = Replace Array Subset(array=w30, new element=w31, index=6) -> (w29:u8[])
            n451 = Greater Than 0?(x=w44) -> (x > 0?=w43:bool)
          }
          frame 1, Default {
            n452 = Delete From Array(array=w56, length=14 ("index"), index=0 ("length")) -> (deleted portion=w49:u8[], array with subset deleted=w60:u8[])
            n453 = Array Size(array=w56) -> (size(s)=w55:i32)
            n454 = Array Size(array=w60) -> (size(s)=w59:i32)
            n455 = Replace Array Subset(array=w50, new element=w49, index=1) -> (w52:u8[])
            n456 = Greater?(x=w55, y=13 ("index")) -> (0:w54:bool)
            n457 = Greater Than 0?(x=w59) -> (x > 0?=w57:bool)
            n458 = Or(x=w54, y=w57) -> (x .or. y?=w58:bool)
          }
        }
      }
      n459 = Transpose 2D Array(2D array=w12) -> (transposed array=→"Downlink":u8[][])
    }
    frame Error {
    }
  }
  "error out" <- w2
  n460 = disable-structure shown="Enabled" {
    frame Disabled {
    }
    frame Enabled {
    }
  }
